vi "AmplifierPowerTest.vi"() -> ()   [LabVIEW 2020]
uses:
  FunctionVi/Window/Control/Channel.ctl
  FunctionVi/Queue/Control/QueueState.ctl
  FunctionVi/Window/Control/Bit rate.ctl
  FunctionVi/Window/Control/HwType.ctl
  FunctionVi/Window/Control/Mode.ctl
  <vilib>/Utility/xml.llb/Read From XML File(string).vi
  <vilib>/Utility/file.llb/Write Delimited Spreadsheet (string).vi
  <vilib>/Utility/xml.llb/Read From XML File(array).vi
  <vilib>/Utility/xml.llb/Write to XML File(string).vi
  <userlib>/FTLDCPower/MPD.lvlib
  <userlib>/PCAN-Basic/PCANBasic.lvlib
  FunctionVi/Window/Win_PowerAmplifier_Transmit.vi
panel:
  in  "USB Config":bool
  out "Interface Information: 3":string
  out "Elapsed Time (s)":dbl caption="已用时间(s)"
  out "Interface Information: 2":string
  in  "HostOCPEnable":bool
  in  "Host OCP":dbl caption="OCP:" format="%#.3gA"
  in  "HostOVPEnable":bool
  in  "Host OVP":dbl caption="OVP:" format="%#.3gV"
  in  "Host Current":dbl caption="Current:" format="%#.3gA"
  in  "Host Voltage":dbl caption="Voltage:" min=0.0 max=45.0 format="%#.3gV"
  out "Host Voltage out":dbl caption="Measure Voltage" format="%#.3gV"
  out "Host Power out":dbl caption="Measure Power" format="%#.3gW"
  out "Host Current out":dbl caption="Measure Current" format="%#.3gA"
  in  "Pause next(ms)":dbl=10.0 caption="Pause next:" min=10.0 format="%#.2fms"
  in  "Pause up(ms)":dbl=10.0 caption="Pause up:" format="%#.3fms"
  in  "ExecuteTime(s)":dbl=5.0 caption="Execute:" min=1.0 format="%#.3gs"
  out "x-y":u32
  out "Status":bool
  out "Company:":string
  out "Time:":string
  out "Channel:":T1 items=["PCAN_USBBUS1"=81, "PCAN_USBBUS2"=82, "PCAN_USBBUS3"=83, "PCAN_USBBUS4"=84]
  in  "PCAN Read error":string
  in  "source":string
  out "Status:":string
  out "Interface Information:":string
  in  "Max voltage":dbl
  in  "At voltage":dbl
  in  "List record":i32(listbox)
  in  "Reset":bool
  in  "指示灯":bool
  in  "On/Off":bool
  in  "ACCOCPEnable":bool
  in  "ACC OCP":dbl caption="OCP:" format="%#.3gA"
  in  "ACCOVPEnable":bool
  in  "ACC OVP":dbl caption="OVP:" format="%#.3gV"
  in  "ACC Current":dbl caption="Current:" min=0.0 format="%#.3gA"
  in  "ACC Voltage":dbl caption="Voltage:" min=0.0 max=45.0 format="%#.3gV"
  in  "Transmit info":bool
  in  "Receive":i32(listbox)
  out "LastError":string
  in  "PCAN Config":bool
  out "ACC Voltage out":dbl caption="Measure Voltage" format="%#.3gV"
  out "ACC Power out":dbl caption="Measure Power" format="%#.3gW"
  out "ACC Current out":dbl caption="Measure Current" format="%#.3gA"
  in  "RS232 Config":bool
  # "ACC Power"
  # "Host Power"
  # "Params Set"
  # "Measurement"
  # "Time"
  # "Output"
  # "Params Set"
  # "Measurement"
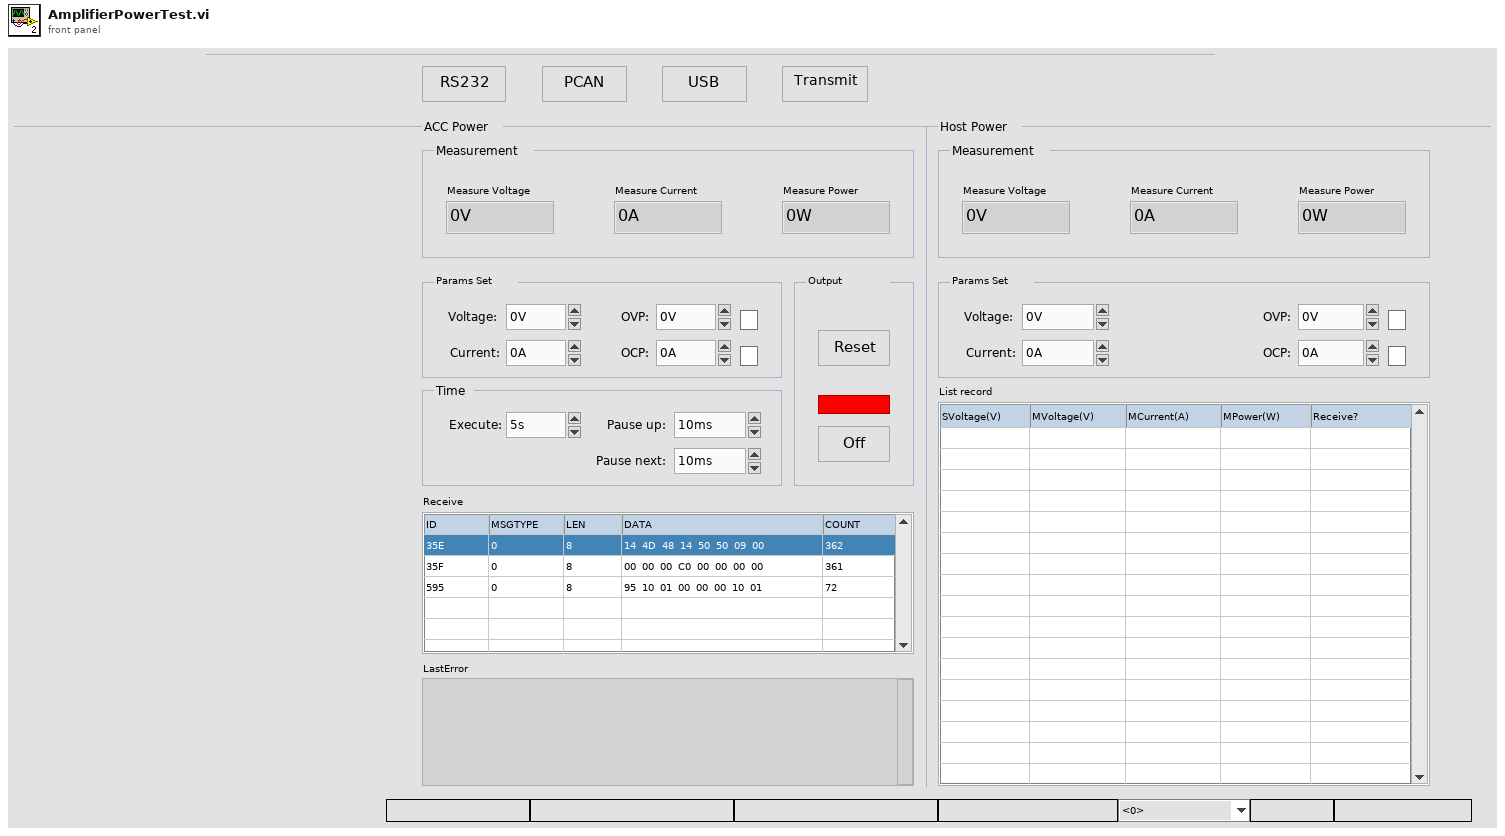
[diagram p1: front panel]
types:
  T1 = typedef "Channel.ctl" = u16
  T2 = typedef "QueueState.ctl" = enum16{"", "Create", "In", "Out", "Empty", "Close"}
  T3 = cluster{"ID":u32, "MSGTYPE":u8, "LEN":u8, "DATA[0]":u8, "DATA[1]":u8, "DATA[2]":u8, "DATA[3]":u8, "DATA[4]":u8, "DATA[5]":u8, "DATA[6]":u8, "DATA[7]":u8}
  T4 = enum8{"Enabled", "Disabled", "Disabled and Grayed Out"}
  T5 = cluster{"ACCCommName":refnum<visa-resource-name>, "HostCommName":refnum<visa-resource-name>}
  T6 = cluster{"ACC Serial Configuration":cluster{"Baud Rate":u32, "Parity":u16, "Data Bits":u16, "Stop Bits":u16, "Flow Control":u16}, "Host ACC Serial Configuration":cluster{"Baud Rate":u32, "Parity":u16, "Data Bits":u16, "Stop Bits":u16, "Flow Control":u16}}
  T7 = typedef "Mode.ctl" = u8
  T8 = typedef "Bit rate.ctl" = u16
  T9 = typedef "HwType.ctl" = u8
  T10 = enum16{"VOLTage", "DEFault", "MINimum", "MAXimum"}
  T11 = cluster{"Baud Rate":u32, "Parity":u16, "Data Bits":u16, "Stop Bits":u16, "Flow Control":u16}
  T12 = enum16{"current", "DEFault", "MINimum", "MAXimum"}
  T13 = typedef "LVPoint32TypeDef.ctl" = cluster{"Horizontal":i32, "Vertical":i32}
  T14 = typedef "LVRowAndColumnTypeDef.ctl" = cluster{"Row":i32, "Column":i32}
  T15 = cluster{"ID":u32, "MSGTYPE":u8, "LEN":u8, "DATA[0]":u8, "DATA[1]":u8, "DATA[2]":u8, "DATA[3]":u8, "DATA[4]":u8, "DATA[5]":u8, "DATA[6]":u8, "DATA[7]":u8}[]
  T16 = cluster{"Time":u16, "MessageBuffer":cluster{"ID":u32, "MSGTYPE":u8, "LEN":u8, "DATA[0]":u8, "DATA[1]":u8, "DATA[2]":u8, "DATA[3]":u8, "DATA[4]":u8, "DATA[5]":u8, "DATA[6]":u8, "DATA[7]":u8}[]}[]
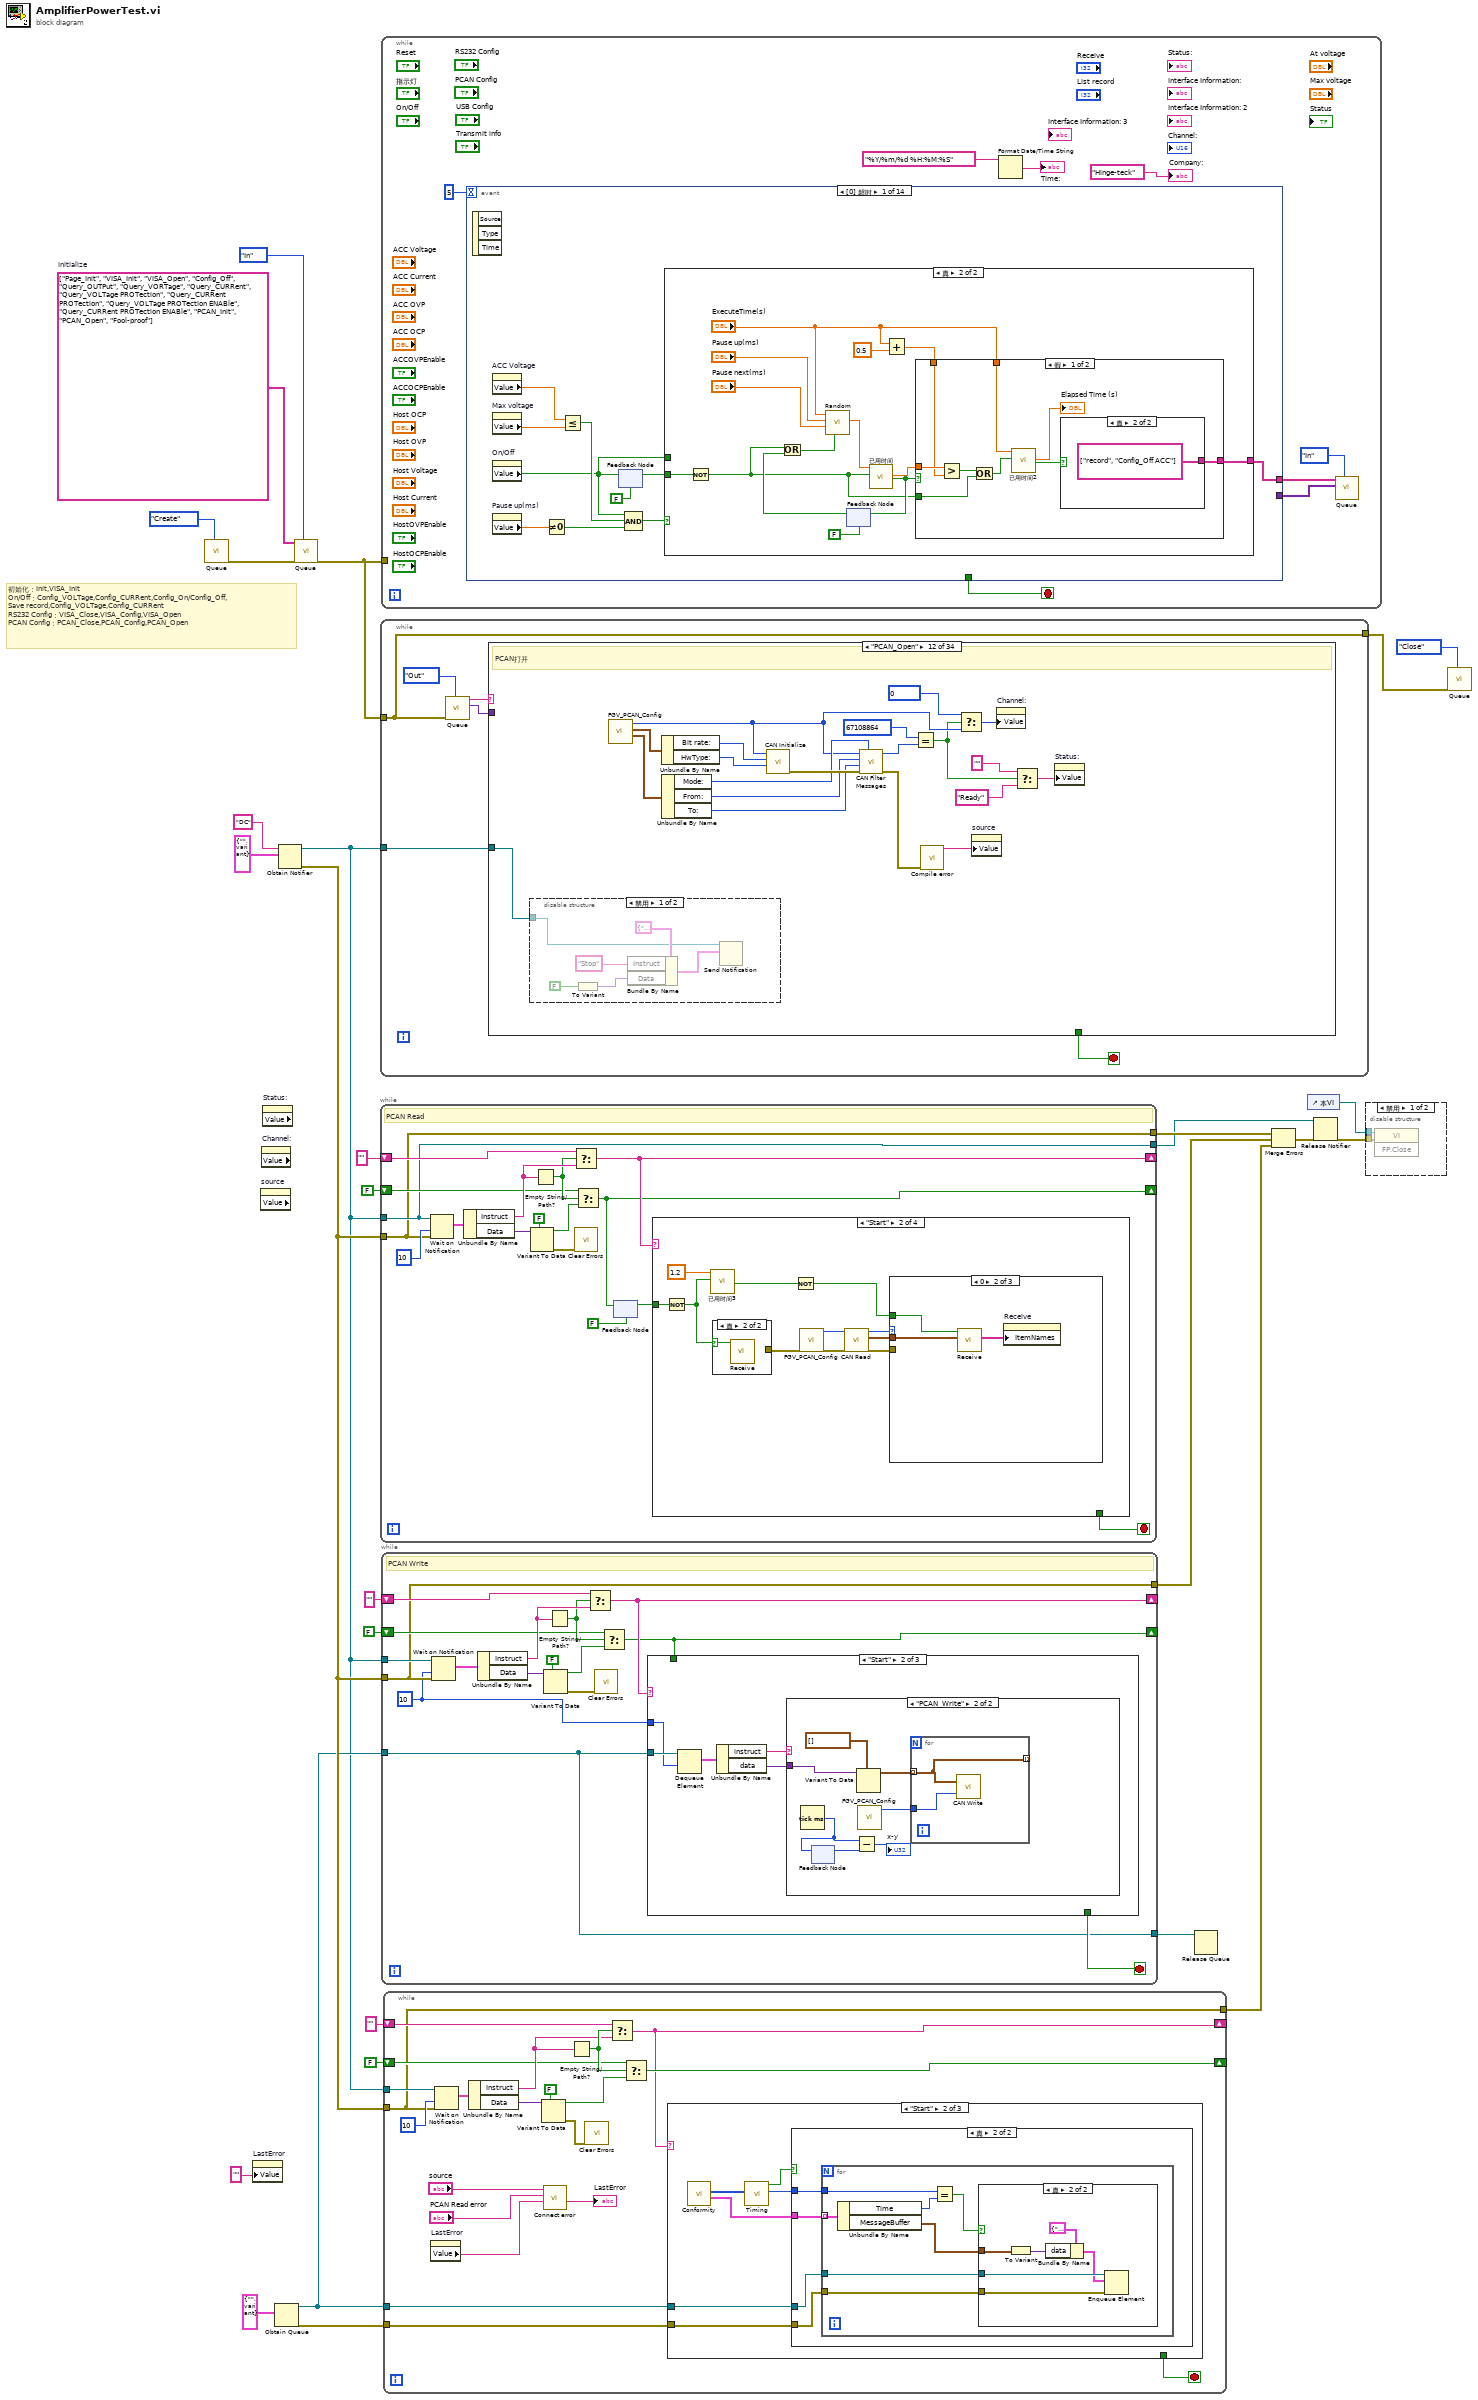
[diagram p0: block diagram]
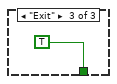
[diagram p6: hidden frame]
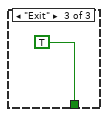
[diagram p9: hidden frame]
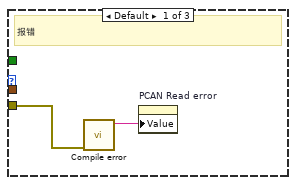
[diagram p11: hidden frame]
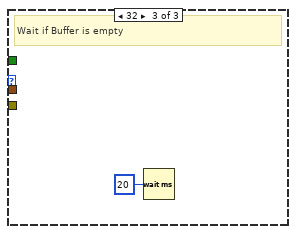
[diagram p12: hidden frame]
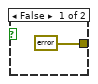
[diagram p13: hidden frame]
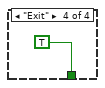
[diagram p15: hidden frame]
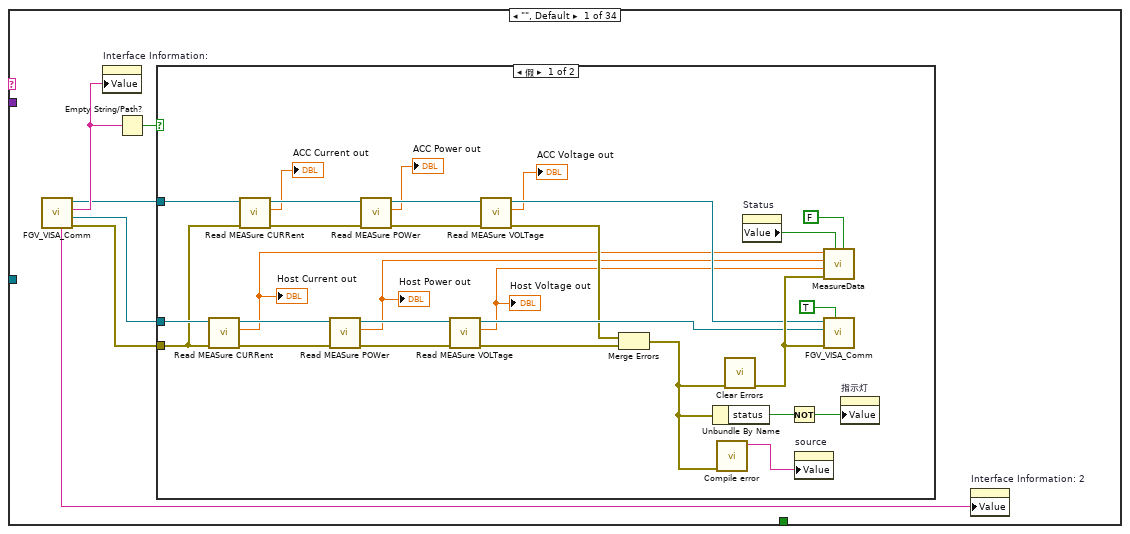
[diagram p16: hidden frame]
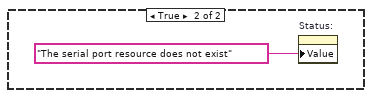
[diagram p17: hidden frame]
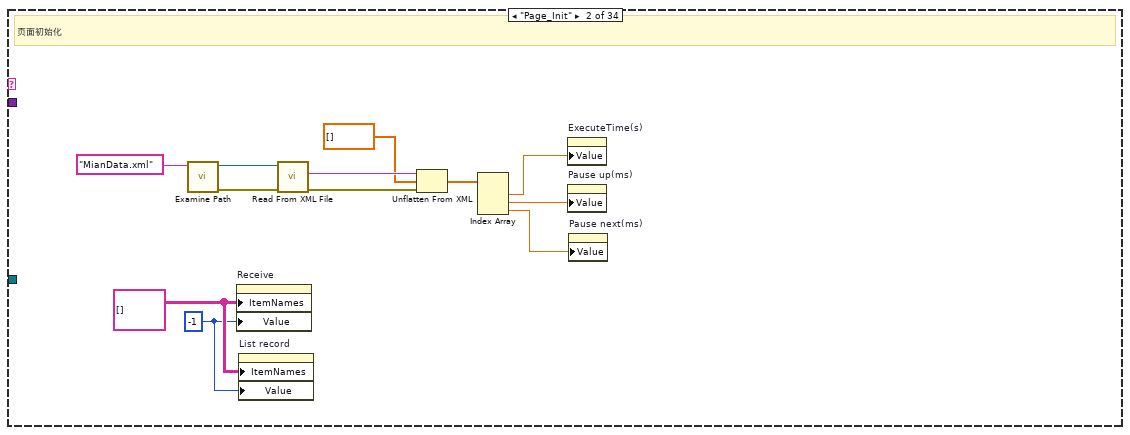
[diagram p18: hidden frame]
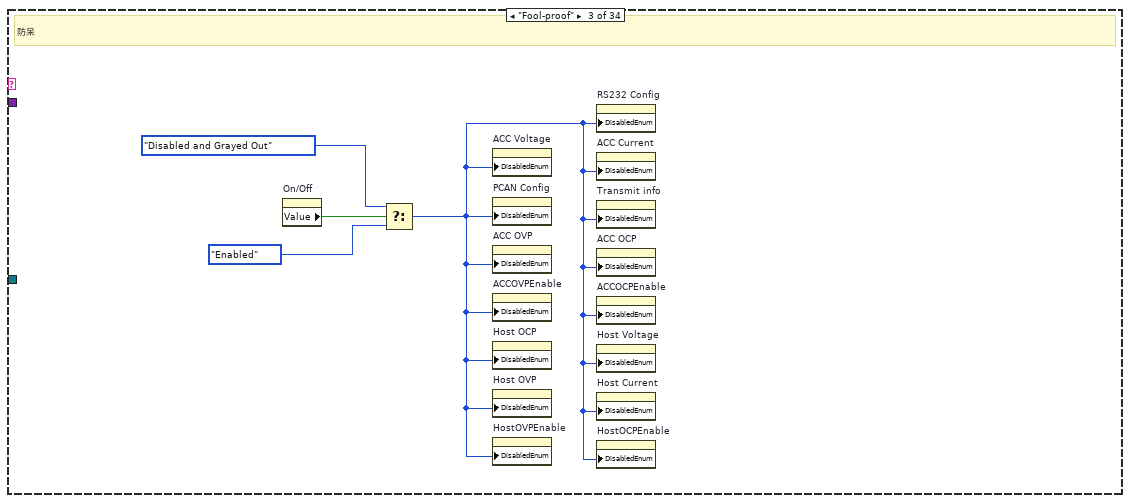
[diagram p19: hidden frame]
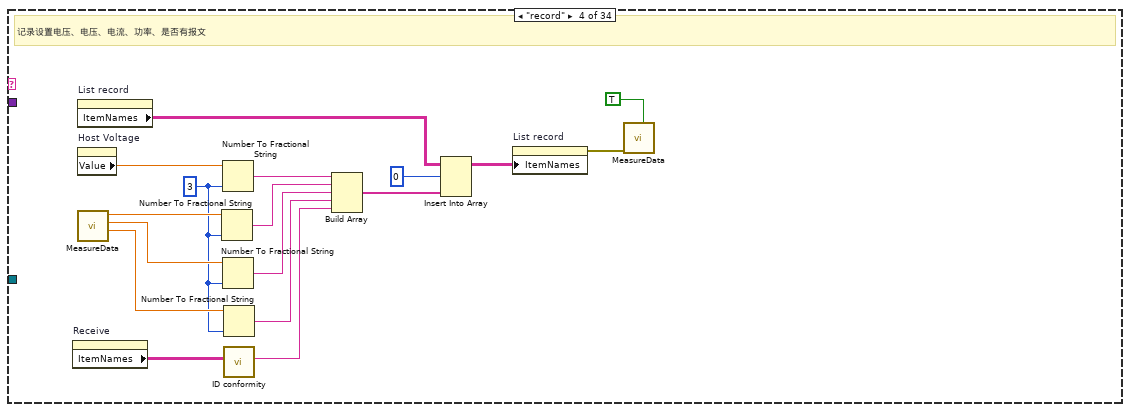
[diagram p20: hidden frame]
diagram:
  w25 = string[] ["Page_Init", "VISA_Init", "VISA_Open", "Config_Off", "Query_OUTPut", "Query_VORTage", "Query_CURRent", "Query_VOLTage PROTection", "Query_CURRent PROTection", "Query_VOLTage PROTection ENABle", "Query_CURRent PROTection ENABle", "PCAN_Init", "PCAN_Open", "Fool-proof"]  # Initialize
  # "初始化：Init,VISA_Init\nOn/Off：Config_VOLTage,Config_CURRent,Config_On/Config_Off,\nSave record,Config_VOLTage,Config_CURRent\nRS232 Config：VISA_Close,VISA_Config,VISA_Open\nPCAN Config：PCAN_Close,PCAN_Config,PCAN_Open"
  n1 = call "Queue.vi"("State"=QueueState."Create") -> ("error out"=w28:errorcluster)  [unwired: 8 in, 2 out]
  n2 = property on="LastError" class="Str"("Value"="") -> ()  [unwired: 2 in, 2 out]
  n3 = property on="source" class="Str" props=["Value"]() -> ()  [unwired: 2 in, 3 out]
  n4 = property on="Channel:" class="Ring (严格)" props=["Value"]() -> ()  [unwired: 2 in, 3 out]
  n5 = property on="Status:" class="Str" props=["Value"]() -> ()  [unwired: 2 in, 3 out]
  n6 = Obtain Queue(element data type=cluster{"instruct":string, "data":variant} {"instruct"="", "data"=variant}) -> (queue out=w19:refnum<queue>, error out=w6:errorcluster)  [unwired: 4 in, 1 out]
  n7 = Obtain Notifier(name (unnamed)="DC" ("名称（未命名）"), notification data type=cluster{"Instruct":string, "Data":variant} {"Instruct"="", "Data"=variant}) -> (notifier out=w18:refnum<notifier>, error out=w20:errorcluster)  [unwired: 2 in, 1 out]
  n8 = call "Queue.vi"("State"=QueueState."In", "error in"=w28, "Instruct"=w25) -> ("error out"=w27:errorcluster)  [unwired: 6 in, 2 out]
  n9 = while {
    tunnel: w20 -> [w30]
    tunnel: w18 -> [w35]
    shift-right: [w37] -> _
    shift-left: "" ("Instruct") -> [w43]
    shift-right: [w33] -> _
    shift-left: FALSE -> [w38]
    tunnel: [w35] -> w12
    tunnel: [w30] -> w14
    stop <- w36 stop-if-true
    # "PCAN Read"
    n10 = Wait on Notification(notifier=w35, timeout in ms (-1)=10 ("超时毫秒(-1)"), error in (no error)=w30) -> (notification=w45:cluster{"Instruct":string, "Data":variant})  [unwired: 1 in, 3 out]
    n11 = Unbundle By Name(w45) -> ("Instruct"=w44:string, "Data"=w41:variant)
    n12 = Variant To Data(type=FALSE, Variant=w41) -> (data=w39:bool, error out=w34:errorcluster)  [unwired: 1 in]
    n13 = Empty String/Path?(string/path=w44) -> (empty?=w42:bool)
    n14 = Select(t=w43, s=w42, f=w44) -> (s? t:f=w37:string)
    n15 = call <vilib>:"Clear Errors.vi"("error in (no error)"=w34) -> ()  [unwired: 5 in, 2 out]
    n16 = Select(t=w38, s=w42, f=w39) -> (s? t:f=w33:bool)
    n17 = feedback-in #1(w33) -> ()
    n18 = feedback #1(FALSE) -> (w31:bool)
    n19 = case shown="\"Start\"" w37 {
      tunnel: [_ _ _ TRUE] -> w36
      tunnel: w31 -> [_ w57 _ _]
      frame "假", Default {
      }
      frame "Start" {
        n20 = Not(x=w57) -> (.not. x?=w55:bool)
        n21 = call "已用时间3"("Time Target (s)"=1.2, "Reset"=w55) -> ("Time has Elapsed"=w48:bool)  [unwired: 10 in, 7 out]
        n22 = case shown="真" w55 {
          selector: w55 -> [_ w65]
          tunnel: [errorcluster {"status"=FALSE, "code"=0, "source"=""} ("错误常量") _] -> w56
          frame False {
          }
          frame True {
            n23 = call "Receive.vi"("Clear?"=w65) -> ()  [unwired: 10 in, 1 out]
          }
        }
        n24 = Not(x=w48) -> (.not. x?=w47:bool)
        n25 = call "FGV_PCAN_Config.vi"("error in"=w56) -> ("error out"=w51:errorcluster, "Channel out"=w53:T1)  [unwired: 7 in, 2 out]
        n26 = call <userlib>:"CAN Read.vi"("error in (no error)"=w51, "Channel"=w53) -> ("error out"=w50:errorcluster, "MessageBuffer out"=w49:T3, "function return"=w52:u32)  [unwired: 6 in, 1 out]
        n27 = case shown="0" w52 {
          tunnel: w50 -> [w59 _ _]
          tunnel: w49 -> [_ w62 _]
          tunnel: w47 -> [_ w60 _]
          frame Default {
            # "报错"
            n28 = call "Compile error.vi"("错误输入"=w59) -> ("Error out"=w58:string)  [unwired: 10 in]
            n29 = property on="PCAN Read error" class="Str"("Value"=w58) -> ()  [unwired: 2 in, 2 out]
          }
          frame 0 {
            n30 = call "Receive.vi"("MessageBuffer"=w62, "Clear?"=w60) -> ("Receive"=w61:string[][])  [unwired: 9 in]
            n31 = property on="Receive" class="MCListbox (严格)"("ItemNames"=w61) -> ()  [unwired: 2 in, 2 out]
          }
          frame 32 {
            # "Wait if Buffer is empty"
            n32 = Wait (ms)(milliseconds to wait=u32 20 ("等待时间（毫秒）")) -> ()  [unwired: 1 out]
          }
        }
      }
      frame "Stop" {
      }
      frame "Exit" {
      }
    }
  }
  n33 = while {
    tunnel: w27 -> [w68]
    tunnel: w18 -> [w67]
    tunnel: [w68] -> w22
    stop <- w70 stop-if-true
    n34 = call "Queue.vi"("State"=QueueState."Out", "error in"=w68) -> ("Data Out"=w69:variant, "Instruct Out"=w71:string)  [unwired: 7 in, 1 out]
    n35 = case shown="\"PCAN_Open\"" w71 {
      tunnel: [_ _ _ _ _ _ _ _ _ _ _ _ _ _ _ _ _ _ _ _ _ _ _ _ _ _ _ _ _ _ _ _ _ TRUE] -> w70
      tunnel: w69 -> [_ _ _ _ _ _ _ _ _ _ _ _ _ _ _ w280 _ _ _ _ _ _ _ _ _ _ _ _ _ _ _ _ _ _]
      tunnel: w67 -> [_ _ _ _ _ _ _ _ _ _ _ w236 _ _ _ _ _ _ _ _ _ w361 w375 w390 w406 w441 _ _ _ _ _ _ _ w548]
      frame "", Default {
        n36 = call "FGV_VISA_Comm.vi"() -> ("error out"=w78:errorcluster, "Host VISA resource name out"=w74:refnum<visa-resource-name>, "ACC Interface Information"=w76:string, "ACC VISA resource name out"=w73:refnum<visa-resource-name>, "Host Interface Information"=w75:string)  [unwired: 7 in]
        n37 = property on="Interface Information:" class="Str"("Value"=w76) -> ()  [unwired: 2 in, 2 out]
        n38 = Empty String/Path?(string/path=w76) -> (empty?=w77:bool)
        n39 = case shown="假" w77 {
          tunnel: w78 -> [w93 _]
          tunnel: w74 -> [w103 _]
          tunnel: w73 -> [w92 _]
          frame False {
            n40 = call <userlib>:"Read MEASure CURRent.vi"("error in (no error)"=w93, "VISA resource name"=w103) -> ("error out"=w107:errorcluster, "Measure Current"=w84:dbl, "VISA resource name out"=w104:refnum<visa-resource-name>)  [unwired: 7 in]
            "Host Current out" <- w84
            n41 = call <userlib>:"Read MEASure CURRent.vi"("error in (no error)"=w93, "VISA resource name"=w92) -> ("error out"=w94:errorcluster, "Measure Current"=→"ACC Current out":dbl, "VISA resource name out"=w91:refnum<visa-resource-name>)  [unwired: 7 in]
            n42 = call <userlib>:"Read MEASure POWer.vi"("error in (no error)"=w107, "VISA resource name"=w104) -> ("error out"=w105:errorcluster, "Measure Power"=w83:dbl, "VISA resource name out"=w106:refnum<visa-resource-name>)  [unwired: 7 in]
            "Host Power out" <- w83
            n43 = call <userlib>:"Read MEASure POWer.vi"("error in (no error)"=w94, "VISA resource name"=w91) -> ("error out"=w95:errorcluster, "Measure Power"=→"ACC Power out":dbl, "VISA resource name out"=w90:refnum<visa-resource-name>)  [unwired: 7 in]
            n44 = call <userlib>:"Read MEASure VOLTage.vi"("error in (no error)"=w105, "VISA resource name"=w106) -> ("error out"=w87:errorcluster, "Measure VOLTage"=w82:dbl, "VISA resource name out"=w88:refnum<visa-resource-name>)  [unwired: 7 in]
            "Host Voltage out" <- w82
            n45 = call <userlib>:"Read MEASure VOLTage.vi"("error in (no error)"=w95, "VISA resource name"=w90) -> ("error out"=w86:errorcluster, "Measure VOLTage"=→"ACC Voltage out":dbl, "VISA resource name out"=w89:refnum<visa-resource-name>)  [unwired: 7 in]
            n46 = Merge Errors(w86, w87) -> (w85:errorcluster)
            n47 = Unbundle By Name(w85) -> ("status"=w101:bool)
            n48 = call "Compile error.vi"("错误输入"=w85) -> ("Error out"=w98:string)  [unwired: 10 in]
            n49 = call <vilib>:"Clear Errors.vi"("error in (no error)"=w85) -> ("error out"=w99:errorcluster)  [unwired: 5 in, 1 out]
            n50 = property on="Status" class="Bool (严格)"() -> ("Value"=w97:bool)  [unwired: 2 in, 2 out]
            n51 = Not(x=w101) -> (.not. x?=w100:bool)
            n52 = property on="source" class="Str"("Value"=w98) -> ()  [unwired: 2 in, 2 out]
            n53 = call "MeasureData.vi"("Reset?"=FALSE, "Write?"=w97, "error in"=w99, "Measure Voltage"=w82, "Measure Power"=w83, "Measure Current"=w84) -> ()  [unwired: 2 in, 4 out]
            n54 = call "FGV_VISA_Comm.vi"("Write?"=TRUE, "error in"=w99, "Host VISA resource name"=w88, "ACC VISA resource name"=w89) -> ()  [unwired: 3 in, 5 out]
            n55 = property on="指示灯" class="Bool (严格)"("Value"=w100) -> ()  [unwired: 2 in, 2 out]
          }
          frame True {
            n56 = property on="Status:" class="Str"("Value"="The serial port resource does not exist") -> ()  [unwired: 2 in, 2 out]
          }
        }
        n57 = property on="Interface Information: 2" class="Str"("Value"=w75) -> ()  [unwired: 2 in, 2 out]
      }
      frame "Page_Init" {
        w119 = -1 ("Receive")
        w120 = string[][] [] ("项名")
        # "页面初始化"
        n58 = call "Examine Path.vi"("Filename"="MianData.xml") -> ("error out"=w116:errorcluster, "Path"=w117:path)  [unwired: 9 in]
        n59 = property on="Receive" class="MCListbox (严格)"("ItemNames"=w120, "Value"=w119) -> ()  [unwired: 2 in, 2 out]
        n60 = property on="List record" class="MCListbox (严格)"("ItemNames"=w120, "Value"=w119) -> ()  [unwired: 2 in, 2 out]
        n61 = call-poly <vilib>:"Read From XML File.vi"("error in (no error)"=w116, "XML File Path"=w117) -> ("error out"=w114:errorcluster, "XML Elements"=w115:string)  [unwired: 7 in, 1 out]
        n62 = Unflatten From XML(xml string=w115, type=dbl[] [], error in (no error)=w114) -> (value=w112:dbl[])  [unwired: 1 out]
        n63 = Index Array(array=w112) -> (element #1=w111:dbl, element #2=w110:dbl, element #3=w109:dbl)  [unwired: 3 in]
        n64 = property on="ExecuteTime(s)" class="DigNum (严格)"("Value"=w111) -> ()  [unwired: 2 in, 2 out]
        n65 = property on="Pause up(ms)" class="DigNum (严格)"("Value"=w110) -> ()  [unwired: 2 in, 2 out]
        n66 = property on="Pause next(ms)" class="DigNum (严格)"("Value"=w109) -> ()  [unwired: 2 in, 2 out]
      }
      frame "Fool-proof" {
        # "防呆"
        n67 = property on="On/Off" class="Bool (严格)"() -> ("Value"=w124:bool)  [unwired: 2 in, 2 out]
        n68 = Select(t=T4."Disabled and Grayed Out" ("禁用"), s=w124, f=T4."Enabled") -> (s? t:f=w121:T4)
        n69 = property on="ACC Voltage" class="DigNum (严格)"("DisabledEnum"=w121) -> ()  [unwired: 2 in, 2 out]
        n70 = property on="PCAN Config" class="Bool"("DisabledEnum"=w121) -> ()  [unwired: 2 in, 2 out]
        n71 = property on="ACC OVP" class="DigNum (严格)"("DisabledEnum"=w121) -> ()  [unwired: 2 in, 2 out]
        n72 = property on="ACCOVPEnable" class="Bool (严格)"("DisabledEnum"=w121) -> ()  [unwired: 2 in, 2 out]
        n73 = property on="Host OCP" class="DigNum (严格)"("DisabledEnum"=w121) -> ()  [unwired: 2 in, 2 out]
        n74 = property on="Host OVP" class="DigNum (严格)"("DisabledEnum"=w121) -> ()  [unwired: 2 in, 2 out]
        n75 = property on="HostOVPEnable" class="Bool (严格)"("DisabledEnum"=w121) -> ()  [unwired: 2 in, 2 out]
        n76 = property on="RS232 Config" class="Bool"("DisabledEnum"=w121) -> ()  [unwired: 2 in, 2 out]
        n77 = property on="ACC Current" class="DigNum (严格)"("DisabledEnum"=w121) -> ()  [unwired: 2 in, 2 out]
        n78 = property on="Transmit info" class="Bool"("DisabledEnum"=w121) -> ()  [unwired: 2 in, 2 out]
        n79 = property on="ACC OCP" class="DigNum (严格)"("DisabledEnum"=w121) -> ()  [unwired: 2 in, 2 out]
        n80 = property on="ACCOCPEnable" class="Bool (严格)"("DisabledEnum"=w121) -> ()  [unwired: 2 in, 2 out]
        n81 = property on="Host Voltage" class="DigNum (严格)"("DisabledEnum"=w121) -> ()  [unwired: 2 in, 2 out]
        n82 = property on="Host Current" class="DigNum (严格)"("DisabledEnum"=w121) -> ()  [unwired: 2 in, 2 out]
        n83 = property on="HostOCPEnable" class="Bool (严格)"("DisabledEnum"=w121) -> ()  [unwired: 2 in, 2 out]
      }
      frame "record" {
        w126 = i16 3 ("精度(6)")
        # "记录设置电压、电压、电流、功率、是否有报文"
        n84 = property on="Receive" class="MCListbox (严格)"() -> ("ItemNames"=w141:string[][])  [unwired: 2 in, 2 out]
        n85 = property on="List record" class="MCListbox (严格)"() -> ("ItemNames"=w135:string[][])  [unwired: 2 in, 2 out]
        n86 = property on="Host Voltage" class="DigNum (严格)"() -> ("Value"=w125:dbl)  [unwired: 2 in, 2 out]
        n87 = call "MeasureData.vi"() -> ("PowerAverage(..10)"=w129:dbl, "CurrentAverage(..10)"=w130:dbl, "VoltageAverage(..10)"=w131:dbl)  [unwired: 8 in, 1 out]
        n88 = Number To Fractional String(number=w131, precision (6)=w126) -> (F-format string=w139:string)  [unwired: 2 in]
        n89 = Number To Fractional String(number=w125, precision (6)=w126) -> (F-format string=w140:string)  [unwired: 2 in]
        n90 = Number To Fractional String(number=w130, precision (6)=w126) -> (F-format string=w138:string)  [unwired: 2 in]
        n91 = Number To Fractional String(number=w129, precision (6)=w126) -> (F-format string=w137:string)  [unwired: 2 in]
        n92 = call "ID conformity.vi"("项名"=w141) -> ("ID conformity"=w136:string)  [unwired: 10 in]
        n93 = Build Array(w140, w139, w138, w137, w136) -> (w134:string[])
        n94 = Insert Into Array(array=w135, index (row)=0 ("索引 (行)"), new element=w134) -> (w132:string[][])  [unwired: 1 in]
        n95 = property on="List record" class="MCListbox (严格)"("ItemNames"=w132) -> (error out=w128:errorcluster)  [unwired: 2 in, 1 out]
        n96 = call "MeasureData.vi"("Reset?"=TRUE, "error in"=w128) -> ()  [unwired: 6 in, 4 out]
      }
      frame "Save record" {
        n97 = Format Date/Time String(time format string (%c)="%Y-%m-%d %H-%M-%S" ("时间格式字符串(%c)")) -> (date/time string=w155:string)  [unwired: 2 in]
        n98 = call <vilib>:"Application Directory.vi"() -> ("Application Directory"=w158:path)
        n99 = Concatenate Strings("Data\\" ("字符串"), w155, " List record.csv" ("字符串")) -> (w153:string)
        n100 = property on="List record" class="MCListbox (严格)"() -> ("ItemNames"=w143:string[][], "ColHdrString"=w152:string[])  [unwired: 2 in, 2 out]
        n101 = Build Path(base path=w158, name or relative path=w153) -> (appended path=w144:path)
        n102 = Strip Path(path=w144) -> (stripped path=w149:path)  [unwired: 1 out]
        n103 = call <vilib>:"Check if File or Folder Exists.vi"("path"=w149) -> ("error out"=w146:errorcluster, "file or folder exists?"=w148:bool, "dup path"=w147:path)  [unwired: 8 in]
        n104 = Empty Array?(array=w143) -> (empty?=w142:bool)
        n105 = Insert Into Array(array=w143, index (row)=0 ("索引 (行)"), new element=w152) -> (w150:string[][])  [unwired: 1 in]
        n106 = case shown="真" w148 {
          tunnel: w147 -> [w165 _]
          tunnel: w146 -> [w164 w166]
          tunnel: [w163 w166] -> w145
          frame False {
            n107 = Create Folder(path (use dialog)=w165, error in=w164) -> (error out=w163:errorcluster)  [unwired: 1 in, 2 out]
          }
          frame True {
          }
        }
        n108 = case shown="真" w142 {
          tunnel: w150 -> [w161 _]
          tunnel: w145 -> [w160 _]
          tunnel: w144 -> [w159 _]
          frame False {
            n109 = call-poly <vilib>:"Write Delimited Spreadsheet.vi"("file path (dialog if empty)"=w159, "2D data"=w161, "error in (no error)"=w160, "delimiter (\\t)"="," ("delimiter (\\t)")) -> ()  [unwired: 10 in, 2 out]
          }
          frame True {
          }
        }
      }
      frame "VISA_Init" {
        # "VISA初始化"
        n110 = call "Examine Path.vi"("Filename"="RS232Data.xml") -> ("error out"=w174:errorcluster, "Path"=w175:path)  [unwired: 9 in]
        n111 = call-poly <vilib>:"Read From XML File.vi"("error in (no error)"=w174, "XML File Path"=w175) -> ("XML Elements"=w173:string[])  [unwired: 7 in, 2 out]
        n112 = Index Array(array=w173) -> (element #1=w172:string, element #2=w171:string)  [unwired: 2 in]
        n113 = Unflatten From XML(xml string=w171, type=T6 {"ACC Serial Configuration"={"Baud Rate"=9600, "Parity"=0, "Data Bits"=8, "Stop Bits"=10, "Flow Control"=0}, "Host ACC Serial Configuration"={"Baud Rate"=9600, "Parity"=0, "Data Bits"=8, "Stop Bits"=10, "Flow Control"=0}} ("Serial Configuration Out")) -> (value=w167:T6)  [unwired: 1 in, 1 out]
        n114 = Unflatten From XML(xml string=w172, type=T5 {"ACCCommName"="COM4", "HostCommName"="COM4"} ("CommNameOut")) -> (value=w168:T5)  [unwired: 1 in, 1 out]
        n115 = call "FGV_VISA_Config.vi"("Write?"=TRUE, "Serial Configuration"=w167, "CommName"=w168) -> ()  [unwired: 6 in, 3 out]
      }
      frame "VISA_Config" {
        # "VISA配置参数"
        n116 = call-by-ref "?"() -> ("Yes out"=w178:bool)  [unwired: 12 in, 3 out]
        n117 = case shown="真" w178 {
          frame False {
          }
          frame True {
            n118 = vi-ref "Win_RS232_Config.vi"() -> (w180:refnum<vi>)
            n119 = invoke class="VI" method="Default Vals.Make Curr Default"(reference=w180) -> (reference out=w179:refnum<vi>)  [unwired: 2 in, 2 out]
            n120 = Close Reference(reference=w179) -> ()  [unwired: 1 in, 1 out]
          }
        }
      }
      frame "VISA_Open" {
        w187 = refnum<visa-resource-name> refnum ("VISA resource name")
        # "VISA连接"
        n121 = call "FGV_VISA_Config.vi"() -> ("error out"=w193:errorcluster, "Serial Configuration Out"=w183:T6, "CommNameOut"=w196:T5)  [unwired: 9 in]
        n122 = Unbundle By Name(w196) -> ("ACCCommName"=w192:refnum<visa-resource-name>, "HostCommName"=w191:refnum<visa-resource-name>)
        n123 = Unbundle By Name(w183) -> ("ACC Serial Configuration"=w182:T11, "Host ACC Serial Configuration"=w181:T11)
        n124 = call <userlib>:"Close.vi"("error in (no error)"=w193, "VISA resource name"=w192) -> ("error out"=w205:errorcluster)  [unwired: 9 in]
        n125 = call <userlib>:"Close.vi"("error in (no error)"=w193, "VISA resource name"=w191) -> ("error out"=w194:errorcluster)  [unwired: 9 in]
        n126 = call <vilib>:"Clear Errors.vi"("error in (no error)"=w205) -> ("error out"=w204:errorcluster)  [unwired: 5 in, 1 out]
        n127 = call <vilib>:"Clear Errors.vi"("error in (no error)"=w194) -> ("error out"=w195:errorcluster)  [unwired: 5 in, 1 out]
        n128 = call <userlib>:"Initialize.vi"("VISA resource name"=w192, "Serial Configuration"=w182, "error in (no error)"=w204) -> ("VISA resource name out"=w199:refnum<visa-resource-name>, "error out"=w190:errorcluster)  [unwired: 6 in]
        n129 = call <userlib>:"Initialize.vi"("VISA resource name"=w191, "Serial Configuration"=w181, "error in (no error)"=w195) -> ("VISA resource name out"=w186:refnum<visa-resource-name>, "error out"=w189:errorcluster)  [unwired: 6 in]
        n130 = Merge Errors(w190, w189) -> (w184:errorcluster)
        n131 = Unbundle By Name(w184) -> ("code"=w202:i32)
        n132 = call "Compile error.vi"("错误输入"=w184) -> ("Error out"=w197:string)  [unwired: 10 in]
        n133 = Equal?(x=w202, y=-1073807343) -> (x = y?=w188:bool)
        n134 = property on="source" class="Str"("Value"=w197) -> ()  [unwired: 2 in, 2 out]
        n135 = Select(t=w187, s=w188, f=w199) -> (s? t:f=w198:refnum<visa-resource-name>)
        n136 = Select(t=w187, s=w188, f=w186) -> (s? t:f=w185:refnum<visa-resource-name>)
        n137 = case shown="真" w188 {
          frame False {
          }
          frame True {
            n138 = call "Queue.vi"("State"=QueueState."Empty") -> ()  [unwired: 8 in, 3 out]
          }
        }
        n139 = call "FGV_VISA_Comm.vi"("Write?"=TRUE, "error in"=w184, "Host VISA resource name"=w185, "ACC VISA resource name"=w198) -> ("error out"=w203:errorcluster)  [unwired: 3 in, 4 out]
        n140 = call <vilib>:"Clear Errors.vi"("error in (no error)"=w203) -> ()  [unwired: 5 in, 2 out]
      }
      frame "VISA_Close" {
        # "VISA关闭连接"
        n141 = call "FGV_VISA_Comm.vi"() -> ("error out"=w208:errorcluster, "Host VISA resource name out"=w207:refnum<visa-resource-name>, "ACC VISA resource name out"=w211:refnum<visa-resource-name>)  [unwired: 7 in, 2 out]
        n142 = call <userlib>:"Close.vi"("error in (no error)"=w208, "VISA resource name"=w211) -> ("error out"=w210:errorcluster)  [unwired: 9 in]
        n143 = call <userlib>:"Close.vi"("error in (no error)"=w208, "VISA resource name"=w207) -> ("error out"=w209:errorcluster)  [unwired: 9 in]
        n144 = call <vilib>:"Clear Errors.vi"("error in (no error)"=w210) -> ()  [unwired: 5 in, 2 out]
        n145 = call <vilib>:"Clear Errors.vi"("error in (no error)"=w209) -> ()  [unwired: 5 in, 2 out]
      }
      frame "PCAN_Init" {
        w219 = T1 81 items=["PCAN_USBBUS1"=81, "PCAN_USBBUS2"=82, "PCAN_USBBUS3"=83, "PCAN_USBBUS4"=84] ("Channel:")
        # "PCAN读取配置"
        n146 = call "Examine Path.vi"("Filename"="PCANData.xml") -> ("error out"=w222:errorcluster, "Path"=w223:path)  [unwired: 9 in]
        n147 = call-poly <vilib>:"Read From XML File.vi"("error in (no error)"=w222, "XML File Path"=w223) -> ("XML Elements"=w221:string[])  [unwired: 7 in, 2 out]
        n148 = call "Examine Path.vi"("Filename"="TransmitData.xml") -> ("error out"=w229:errorcluster, "Path"=w230:path)  [unwired: 9 in]
        n149 = Index Array(array=w221) -> (element #1=w220:string, element #2=w217:string, element #3=w214:string)  [unwired: 3 in]
        n150 = call-poly <vilib>:"Read From XML File.vi"("error in (no error)"=w229, "XML File Path"=w230) -> ("XML Elements"=w228:string)  [unwired: 7 in, 2 out]
        n151 = Unflatten From XML(xml string=w220, type=w219) -> (value=w218:T1)  [unwired: 1 in, 1 out]
        n152 = Unflatten From XML(xml string=w228, type=string[][] []) -> (value=w226:string[][])  [unwired: 1 in, 1 out]
        n153 = Unflatten From XML(xml string=w217, type=cluster{"Bit rate:":T8, "HwType: ":T9} {"Bit rate:"=28, "HwType: "=1} ("Initialize")) -> (value=w215:cluster{"Bit rate:":T8, "HwType: ":T9})  [unwired: 1 in, 1 out]
        n154 = Unflatten From XML(xml string=w214, type=cluster{"Mode: ":T7, "From:":u32, "To:":u32} {"Mode: "=0, "From:"=0, "To:"=0} ("FilterMessages")) -> (value=w212:cluster{"Mode: ":T7, "From:":u32, "To:":u32})  [unwired: 1 in, 1 out]
        n155 = call "FGV_PowerAmplifier_Transmit.vi"("Write?"=TRUE, "Transmit"=w226) -> ()  [unwired: 8 in, 2 out]
        n156 = call "FGV_PCAN_Config.vi"("Write?"=TRUE, "FilterMessages"=w212, "Initialize"=w215, "Channel"=w218) -> ()  [unwired: 4 in, 4 out]
      }
      frame "PCAN_Config" {
        # "PCAN配置"
        n157 = call-by-ref "?"() -> ("Yes out"=w233:bool)  [unwired: 9 in, 6 out]
        n158 = case shown="真" w233 {
          frame False {
          }
          frame True {
            n159 = vi-ref "Win_PCAN_Config.vi"() -> (w235:refnum<vi>)
            n160 = invoke class="VI" method="Default Vals.Make Curr Default"(reference=w235) -> (reference out=w234:refnum<vi>)  [unwired: 2 in, 2 out]
            n161 = Close Reference(reference=w234) -> ()  [unwired: 1 in, 1 out]
          }
        }
      }
      frame "PCAN_Open" {
        w242 = T1 0 items=["PCAN_USBBUS1"=81, "PCAN_USBBUS2"=82, "PCAN_USBBUS3"=83, "PCAN_USBBUS4"=84] ("t")
        # "PCAN打开"
        n162 = disable-structure shown="禁用" {
          disable-tunnel: w236 -> [w256 _]
          frame Disabled {
            n163 = To Variant(anything=FALSE) -> (Variant=w258:variant)
            n164 = Bundle By Name(cluster=cluster{"Instruct":string, "Data":variant} {"Instruct"="", "Data"=variant}, "Instruct"="Stop", "Data"=w258) -> (w261:cluster{"Instruct":string, "Data":variant})
            n165 = Send Notification(notification=w261, notifier=w256) -> ()  [unwired: 1 in, 2 out]
          }
          frame Enabled {
          }
        }
        n166 = call "FGV_PCAN_Config.vi"() -> ("FilterMessages out"=w254:cluster{"Mode: ":T7, "From:":u32, "To:":u32}, "Initialize out"=w255:cluster{"Bit rate:":T8, "HwType: ":T9}, "Channel out"=w243:T1)  [unwired: 8 in, 1 out]
        n167 = Unbundle By Name(w255) -> ("Bit rate:"=w253:T8, "HwType:"=w252:T9)
        n168 = Unbundle By Name(w254) -> ("Mode:"=w250:T7, "From:"=w249:u32, "To:"=w248:u32)
        n169 = call <userlib>:"CAN Initialize.vi"("HwType"=w252, "Btr0Btr1"=w253, "Channel"=w243) -> ("错误输出"=w251:errorcluster)  [unwired: 7 in, 1 out]
        n170 = call <userlib>:"CAN Filter Messages.vi"("Mode"=w250, "error in (no error)"=w251, "ToID"=w248, "FromID"=w249, "Channel"=w243) -> ("error out"=w247:errorcluster, "function return"=w245:u32)  [unwired: 5 in]
        n171 = Equal?(x=u32 67108864, y=w245) -> (x = y?=w240:bool)
        n172 = call "Compile error.vi"("错误输入"=w247) -> ("Error out"=w246:string)  [unwired: 10 in]
        n173 = Select(t=w242, s=w240, f=w243) -> (s? t:f=w241:T1)
        n174 = property on="source" class="Str"("Value"=w246) -> ()  [unwired: 2 in, 2 out]
        n175 = property on="Channel:" class="Ring (严格)"("Value"=w241) -> ()  [unwired: 2 in, 2 out]
        n176 = Select(t="", s=w240, f="Ready") -> (s? t:f=w237:string)
        n177 = property on="Status:" class="Str"("Value"=w237) -> ()  [unwired: 2 in, 2 out]
      }
      frame "PCAN_Close" {
        # "PCAN关闭"
        n178 = call "FGV_PCAN_Config.vi"() -> ("Channel out"=w262:T1)  [unwired: 8 in, 3 out]
        n179 = call <userlib>:"CAN Uninitialize.vi"("Channel"=w262) -> ()  [unwired: 10 in, 1 out]
      }
      frame "Transmit_info" {
        # "报文"
        n180 = call-by-ref "?"() -> ("Yes out"=w263:bool)  [unwired: 12 in, 3 out]
        n181 = case shown="真" w263 {
          frame False {
          }
          frame True {
            n182 = vi-ref "Win_PCAN_Config.vi"() -> (w265:refnum<vi>)
            n183 = invoke class="VI" method="Default Vals.Make Curr Default"(reference=w265) -> (reference out=w264:refnum<vi>)  [unwired: 2 in, 2 out]
            n184 = Close Reference(reference=w264) -> ()  [unwired: 1 in, 1 out]
          }
        }
      }
      frame "Config_VOLTage" {
        # "设置输出电压"
        n185 = call "FGV_VISA_Comm.vi"() -> ("error out"=w272:errorcluster, "Host VISA resource name out"=w273:refnum<visa-resource-name>, "ACC VISA resource name out"=w278:refnum<visa-resource-name>)  [unwired: 7 in, 2 out]
        n186 = property on="Host Voltage" class="DigNum (严格)"() -> ("Value"=w271:dbl)  [unwired: 2 in, 2 out]
        n187 = property on="ACC Voltage" class="DigNum (严格)"() -> ("Value"=w275:dbl)  [unwired: 2 in, 2 out]
        n188 = call <userlib>:"Configure VOLTage LEVel.vi"("VOLTage  Value(V)"=w275, "error in (no error)"=w272, "VOLTage Tab"=T10."VOLTage", "VISA resource name"=w278) -> ("error out"=w269:errorcluster, "VISA resource name out"=w277:refnum<visa-resource-name>)  [unwired: 6 in]
        n189 = call <userlib>:"Configure VOLTage LEVel.vi"("VOLTage  Value(V)"=w271, "error in (no error)"=w272, "VOLTage Tab"=T10."VOLTage", "VISA resource name"=w273) -> ("error out"=w268:errorcluster, "VISA resource name out"=w270:refnum<visa-resource-name>)  [unwired: 6 in]
        n190 = Merge Errors(w269, w268) -> (w267:errorcluster)
        n191 = call "FGV_VISA_Comm.vi"("Write?"=TRUE, "error in"=w267, "Host VISA resource name"=w270, "ACC VISA resource name"=w277) -> ("error out"=w266:errorcluster)  [unwired: 3 in, 4 out]
        n192 = call <vilib>:"Clear Errors.vi"("error in (no error)"=w266) -> ()  [unwired: 5 in, 2 out]
      }
      frame "Config_VOLTage1" {
        # "设置输出电压"
        n193 = disable-structure shown="禁用" {
          disable-tunnel: w280 -> [w283 _]
          frame Disabled {
            n194 = Variant To Data(type=0.0 ("x+y"), Variant=w283) -> (data=w281:dbl)  [unwired: 1 in, 1 out]
            n195 = call "FGV_VISA_Comm.vi"() -> ("error out"=w286:errorcluster, "ACC VISA resource name out"=w288:refnum<visa-resource-name>)  [unwired: 7 in, 3 out]
            n196 = call <userlib>:"Configure VOLTage LEVel.vi"("VOLTage  Value(V)"=w281, "error in (no error)"=w286, "VOLTage Tab"=T10."VOLTage", "VISA resource name"=w288) -> ("error out"=w285:errorcluster, "VISA resource name out"=w287:refnum<visa-resource-name>)  [unwired: 6 in]
            n197 = call "FGV_VISA_Comm.vi"("Write?"=TRUE, "error in"=w285, "ACC VISA resource name"=w287) -> ()  [unwired: 4 in, 5 out]
          }
          frame Enabled {
          }
        }
      }
      frame "Config_CURRent" {
        w296 = T12."current" ("Current Tab")
        # "设置输出电流"
        n198 = call "FGV_VISA_Comm.vi"() -> ("error out"=w298:errorcluster, "Host VISA resource name out"=w295:refnum<visa-resource-name>, "ACC VISA resource name out"=w299:refnum<visa-resource-name>)  [unwired: 7 in, 2 out]
        n199 = property on="ACC Current" class="DigNum (严格)"() -> ("Value"=w297:dbl)  [unwired: 2 in, 2 out]
        n200 = property on="Host Current" class="DigNum (严格)"() -> ("Value"=w290:dbl)  [unwired: 2 in, 2 out]
        n201 = call <userlib>:"Configure CURRent LEVel.vi"("Current  Value(A)"=w297, "error in (no error)"=w298, "Current Tab"=w296, "VISA resource name"=w299) -> ("error out"=w293:errorcluster, "VISA resource name out"=w300:refnum<visa-resource-name>)  [unwired: 6 in]
        n202 = call <userlib>:"Configure CURRent LEVel.vi"("Current  Value(A)"=w290, "Current Tab"=w296, "VISA resource name"=w295) -> ("error out"=w292:errorcluster, "VISA resource name out"=w294:refnum<visa-resource-name>)  [unwired: 7 in]
        n203 = Merge Errors(w293, w292) -> (w291:errorcluster)
        n204 = call "FGV_VISA_Comm.vi"("Write?"=TRUE, "error in"=w291, "Host VISA resource name"=w294, "ACC VISA resource name"=w300) -> ()  [unwired: 3 in, 5 out]
      }
      frame "Config_VOLTage PROTection" {
        w307 = T10."VOLTage" ("VOLTage Tab")
        # "设置输出电压保护阈值"
        n205 = call "FGV_VISA_Comm.vi"() -> ("error out"=w308:errorcluster, "Host VISA resource name out"=w309:refnum<visa-resource-name>, "ACC VISA resource name out"=w311:refnum<visa-resource-name>)  [unwired: 7 in, 2 out]
        n206 = property on="ACC OVP" class="DigNum (严格)"() -> ("Value"=w310:dbl)  [unwired: 2 in, 2 out]
        n207 = property on="Host OVP" class="DigNum (严格)"() -> ("Value"=w306:dbl)  [unwired: 2 in, 2 out]
        n208 = call <userlib>:"Configure VOLTage PROTection LEVel.vi"("VISA resource name"=w309, "VOLTage Tab"=w307, "VOLTage Protection Value(V)"=w306, "error in (no error)"=w308) -> ("VISA resource name out"=w305:refnum<visa-resource-name>, "error out"=w303:errorcluster)  [unwired: 4 in]
        n209 = call <userlib>:"Configure VOLTage PROTection LEVel.vi"("VISA resource name"=w311, "VOLTage Tab"=w307, "VOLTage Protection Value(V)"=w310, "error in (no error)"=w308) -> ("VISA resource name out"=w312:refnum<visa-resource-name>, "error out"=w304:errorcluster)  [unwired: 4 in]
        n210 = Merge Errors(w304, w303) -> (w302:errorcluster)
        n211 = call "FGV_VISA_Comm.vi"("Write?"=TRUE, "error in"=w302, "Host VISA resource name"=w305, "ACC VISA resource name"=w312) -> ()  [unwired: 3 in, 5 out]
      }
      frame "Config_CURRent PROTection" {
        w320 = T12."current" ("Current Tab")
        # "设置输出电流保护阈值"
        n212 = call "FGV_VISA_Comm.vi"() -> ("error out"=w319:errorcluster, "Host VISA resource name out"=w321:refnum<visa-resource-name>, "ACC VISA resource name out"=w323:refnum<visa-resource-name>)  [unwired: 7 in, 2 out]
        n213 = property on="ACC OCP" class="DigNum (严格)"() -> ("Value"=w322:dbl)  [unwired: 2 in, 2 out]
        n214 = property on="Host OCP" class="DigNum (严格)"() -> ("Value"=w318:dbl)  [unwired: 2 in, 2 out]
        n215 = call <userlib>:"Configure CURRent PROTection LEVel.vi"("VISA resource name"=w323, "Current Tab"=w320, "Current Protection Value(A)"=w322, "error in (no error)"=w319) -> ("VISA resource name out"=w324:refnum<visa-resource-name>, "error out"=w316:errorcluster)  [unwired: 4 in]
        n216 = call <userlib>:"Configure CURRent PROTection LEVel.vi"("VISA resource name"=w321, "Current Tab"=w320, "Current Protection Value(A)"=w318, "error in (no error)"=w319) -> ("VISA resource name out"=w317:refnum<visa-resource-name>, "error out"=w315:errorcluster)  [unwired: 4 in]
        n217 = Merge Errors(w316, w315) -> (w314:errorcluster)
        n218 = call "FGV_VISA_Comm.vi"("Write?"=TRUE, "error in"=w314, "Host VISA resource name"=w317, "ACC VISA resource name"=w324) -> ()  [unwired: 3 in, 5 out]
      }
      frame "Config_VOLTage PROTection ENABle" {
        # "禁止或使能当前输出电压保护电路"
        n219 = call "FGV_VISA_Comm.vi"() -> ("error out"=w331:errorcluster, "Host VISA resource name out"=w332:refnum<visa-resource-name>, "ACC VISA resource name out"=w334:refnum<visa-resource-name>)  [unwired: 7 in, 2 out]
        n220 = property on="HostOVPEnable" class="Bool (严格)"() -> ("Value"=w330:bool)  [unwired: 2 in, 2 out]
        n221 = property on="ACCOVPEnable" class="Bool (严格)"() -> ("Value"=w333:bool)  [unwired: 2 in, 2 out]
        n222 = call <userlib>:"Configure VOLTage PROTection ENABle.vi"("error in (no error)"=w331, "Enable VOLTage protection (T: Enable)"=w333, "VISA resource name"=w334) -> ("error out"=w328:errorcluster, "VISA resource name out"=w335:refnum<visa-resource-name>)  [unwired: 7 in]
        n223 = call <userlib>:"Configure VOLTage PROTection ENABle.vi"("error in (no error)"=w331, "Enable VOLTage protection (T: Enable)"=w330, "VISA resource name"=w332) -> ("error out"=w327:errorcluster, "VISA resource name out"=w329:refnum<visa-resource-name>)  [unwired: 7 in]
        n224 = Merge Errors(w328, w327) -> (w326:errorcluster)
        n225 = call "FGV_VISA_Comm.vi"("Write?"=TRUE, "error in"=w326, "Host VISA resource name"=w329, "ACC VISA resource name"=w335) -> ()  [unwired: 3 in, 5 out]
      }
      frame "Config_CURRent PROTection ENABle" {
        # "禁止或使能当前输出电压保护电路"
        n226 = call "FGV_VISA_Comm.vi"() -> ("error out"=w342:errorcluster, "Host VISA resource name out"=w343:refnum<visa-resource-name>, "ACC VISA resource name out"=w345:refnum<visa-resource-name>)  [unwired: 7 in, 2 out]
        n227 = property on="HostOCPEnable" class="Bool (严格)"() -> ("Value"=w341:bool)  [unwired: 2 in, 2 out]
        n228 = property on="ACCOCPEnable" class="Bool (严格)"() -> ("Value"=w344:bool)  [unwired: 2 in, 2 out]
        n229 = call <userlib>:"Configure CURRent PROTection ENABle.vi"("error in (no error)"=w342, "Enable Current protection (T: Enable)"=w344, "VISA resource name"=w345) -> ("error out"=w339:errorcluster, "VISA resource name out"=w346:refnum<visa-resource-name>)  [unwired: 7 in]
        n230 = call <userlib>:"Configure CURRent PROTection ENABle.vi"("error in (no error)"=w342, "Enable Current protection (T: Enable)"=w341, "VISA resource name"=w343) -> ("error out"=w338:errorcluster, "VISA resource name out"=w340:refnum<visa-resource-name>)  [unwired: 7 in]
        n231 = Merge Errors(w339, w338) -> (w337:errorcluster)
        n232 = call "FGV_VISA_Comm.vi"("Write?"=TRUE, "error in"=w337, "Host VISA resource name"=w340, "ACC VISA resource name"=w346) -> ()  [unwired: 3 in, 5 out]
      }
      frame "Config_On" {
        w353 = TRUE ("Enable OUTPut (T: Enable)")
        # "VISA打开通道"
        n233 = To Variant(anything=TRUE) -> (Variant=w356:variant)
        n234 = Bundle By Name(cluster=cluster{"Instruct":string, "Data":variant} {"Instruct"="", "Data"=variant} ("通知"), "Instruct"="Start", "Data"=w356) -> (w359:cluster{"Instruct":string, "Data":variant})
        n235 = call "FGV_VISA_Comm.vi"() -> ("error out"=w352:errorcluster, "Host VISA resource name out"=w354:refnum<visa-resource-name>, "ACC VISA resource name out"=w364:refnum<visa-resource-name>)  [unwired: 7 in, 2 out]
        n236 = Send Notification(notification=w359, notifier=w361) -> ()  [unwired: 1 in, 2 out]
        n237 = call <userlib>:"Configure OUTPut ENABle.vi"("error in (no error)"=w352, "Enable OUTPut (T: Enable)"=w353, "VISA resource name"=w364) -> ("error out"=w350:errorcluster, "VISA resource name out"=w363:refnum<visa-resource-name>)  [unwired: 7 in]
        n238 = call <userlib>:"Configure OUTPut ENABle.vi"("error in (no error)"=w352, "Enable OUTPut (T: Enable)"=w353, "VISA resource name"=w354) -> ("error out"=w349:errorcluster, "VISA resource name out"=w351:refnum<visa-resource-name>)  [unwired: 7 in]
        n239 = Merge Errors(w350, w349) -> (w348:errorcluster)
        n240 = call "FGV_VISA_Comm.vi"("Write?"=TRUE, "error in"=w348, "Host VISA resource name"=w351, "ACC VISA resource name"=w363) -> ()  [unwired: 3 in, 5 out]
        n241 = property on="Status" class="Bool (严格)"("Value"=TRUE ("Status")) -> ()  [unwired: 2 in, 2 out]
      }
      frame "Config_On ACC" {
        # "VISA打开通道"
        n242 = To Variant(anything=TRUE) -> (Variant=w370:variant)
        n243 = Bundle By Name(cluster=cluster{"Instruct":string, "Data":variant} {"Instruct"="", "Data"=variant} ("通知"), "Instruct"="Start", "Data"=w370) -> (w373:cluster{"Instruct":string, "Data":variant})
        n244 = call "FGV_VISA_Comm.vi"() -> ("error out"=w367:errorcluster, "Host VISA resource name out"=w365:refnum<visa-resource-name>, "ACC VISA resource name out"=w378:refnum<visa-resource-name>)  [unwired: 7 in, 2 out]
        n245 = Send Notification(notification=w373, notifier=w375) -> ()  [unwired: 1 in, 2 out]
        n246 = call <userlib>:"Configure OUTPut ENABle.vi"("error in (no error)"=w367, "Enable OUTPut (T: Enable)"=TRUE, "VISA resource name"=w378) -> ("error out"=w366:errorcluster, "VISA resource name out"=w377:refnum<visa-resource-name>)  [unwired: 7 in]
        n247 = call "FGV_VISA_Comm.vi"("Write?"=TRUE, "error in"=w366, "Host VISA resource name"=w365, "ACC VISA resource name"=w377) -> ()  [unwired: 3 in, 5 out]
        n248 = property on="Status" class="Bool (严格)"("Value"=TRUE ("Status")) -> ()  [unwired: 2 in, 2 out]
      }
      frame "Config_Off" {
        w385 = FALSE ("Enable OUTPut (T: Enable)")
        # "VISA关闭通道"
        n249 = To Variant(anything=FALSE) -> (Variant=w391:variant)
        n250 = Bundle By Name(cluster=cluster{"Instruct":string, "Data":variant} {"Instruct"="", "Data"=variant}, "Instruct"="Stop", "Data"=w391) -> (w394:cluster{"Instruct":string, "Data":variant})
        n251 = call "FGV_VISA_Comm.vi"() -> ("error out"=w383:errorcluster, "Host VISA resource name out"=w384:refnum<visa-resource-name>, "ACC VISA resource name out"=w397:refnum<visa-resource-name>)  [unwired: 7 in, 2 out]
        n252 = Send Notification(notification=w394, notifier=w390) -> ()  [unwired: 1 in, 2 out]
        n253 = call <userlib>:"Configure OUTPut ENABle.vi"("error in (no error)"=w383, "Enable OUTPut (T: Enable)"=w385, "VISA resource name"=w397) -> ("error out"=w381:errorcluster, "VISA resource name out"=w396:refnum<visa-resource-name>)  [unwired: 7 in]
        n254 = call <userlib>:"Configure OUTPut ENABle.vi"("error in (no error)"=w383, "Enable OUTPut (T: Enable)"=w385, "VISA resource name"=w384) -> ("error out"=w380:errorcluster, "VISA resource name out"=w382:refnum<visa-resource-name>)  [unwired: 7 in]
        n255 = Merge Errors(w381, w380) -> (w379:errorcluster)
        n256 = call <vilib>:"Clear Errors.vi"("error in (no error)"=w379) -> ("error out"=w388:errorcluster)  [unwired: 5 in, 1 out]
        n257 = call "Compile error.vi"("错误输入"=w379) -> ("Error out"=w387:string)  [unwired: 10 in]
        n258 = property on="source" class="Str"("Value"=w387) -> ()  [unwired: 2 in, 2 out]
        n259 = call "FGV_VISA_Comm.vi"("Write?"=TRUE, "error in"=w388, "Host VISA resource name"=w382, "ACC VISA resource name"=w396) -> ()  [unwired: 3 in, 5 out]
        n260 = property on="Status" class="Bool (严格)"("Value"=FALSE ("Status")) -> ()  [unwired: 2 in, 2 out]
      }
      frame "Config_Off ACC" {
        # "VISA关闭通道"
        n261 = To Variant(anything=FALSE) -> (Variant=w407:variant)
        n262 = Bundle By Name(cluster=cluster{"Instruct":string, "Data":variant} {"Instruct"="", "Data"=variant}, "Instruct"="Stop", "Data"=w407) -> (w410:cluster{"Instruct":string, "Data":variant})
        n263 = Send Notification(notification=w410, notifier=w406) -> ()  [unwired: 1 in, 2 out]
        n264 = call "FGV_VISA_Comm.vi"() -> ("error out"=w400:errorcluster, "Host VISA resource name out"=w398:refnum<visa-resource-name>, "ACC VISA resource name out"=w413:refnum<visa-resource-name>)  [unwired: 7 in, 2 out]
        n265 = call <userlib>:"Configure OUTPut ENABle.vi"("error in (no error)"=w400, "Enable OUTPut (T: Enable)"=FALSE, "VISA resource name"=w413) -> ("error out"=w399:errorcluster, "VISA resource name out"=w412:refnum<visa-resource-name>)  [unwired: 7 in]
        n266 = call <vilib>:"Clear Errors.vi"("error in (no error)"=w399) -> ("error out"=w404:errorcluster)  [unwired: 5 in, 1 out]
        n267 = call "Compile error.vi"("错误输入"=w399) -> ("Error out"=w403:string)  [unwired: 10 in]
        n268 = property on="source" class="Str"("Value"=w403) -> ()  [unwired: 2 in, 2 out]
        n269 = call "FGV_VISA_Comm.vi"("Write?"=TRUE, "error in"=w404, "Host VISA resource name"=w398, "ACC VISA resource name"=w412) -> ()  [unwired: 3 in, 5 out]
        n270 = property on="Status" class="Bool (严格)"("Value"=FALSE ("Status")) -> ()  [unwired: 2 in, 2 out]
      }
      frame "Config_Reset" {
        # "VISA关闭通道、清除保护电路"
        n271 = To Variant(anything=FALSE) -> (Variant=w442:variant)
        n272 = Bundle By Name(cluster=cluster{"Instruct":string, "Data":variant} {"Instruct"="", "Data"=variant}, "Instruct"="Stop", "Data"=w442) -> (w445:cluster{"Instruct":string, "Data":variant})
        n273 = call "FGV_VISA_Comm.vi"() -> ("error out"=w422:errorcluster, "Host VISA resource name out"=w423:refnum<visa-resource-name>, "ACC VISA resource name out"=w448:refnum<visa-resource-name>)  [unwired: 7 in, 2 out]
        n274 = Send Notification(notification=w445, notifier=w441) -> ()  [unwired: 1 in, 2 out]
        n275 = call <userlib>:"Configure OUTPut ENABle.vi"("error in (no error)"=w422, "Enable OUTPut (T: Enable)"=FALSE, "VISA resource name"=w448) -> ("error out"=w438:errorcluster, "VISA resource name out"=w439:refnum<visa-resource-name>)  [unwired: 7 in]
        n276 = call <userlib>:"Configure OUTPut ENABle.vi"("error in (no error)"=w422, "Enable OUTPut (T: Enable)"=FALSE, "VISA resource name"=w423) -> ("error out"=w426:errorcluster, "VISA resource name out"=w425:refnum<visa-resource-name>)  [unwired: 7 in]
        n277 = call <userlib>:"Configure VOLTage PROTection CLEar.vi"("error in (no error)"=w438, "VISA resource name"=w439) -> ("error out"=w436:errorcluster, "VISA resource name out"=w437:refnum<visa-resource-name>)  [unwired: 8 in]
        n278 = call <userlib>:"Configure VOLTage PROTection CLEar.vi"("error in (no error)"=w426, "VISA resource name"=w425) -> ("error out"=w428:errorcluster, "VISA resource name out"=w427:refnum<visa-resource-name>)  [unwired: 8 in]
        n279 = call <userlib>:"Configure CURRent PROTection CLEar.vi"("error in (no error)"=w436, "VISA resource name"=w437) -> ("error out"=w435:errorcluster, "VISA resource name out"=w434:refnum<visa-resource-name>)  [unwired: 8 in]
        n280 = call <userlib>:"Configure CURRent PROTection CLEar.vi"("error in (no error)"=w428, "VISA resource name"=w427) -> ("error out"=w429:errorcluster, "VISA resource name out"=w430:refnum<visa-resource-name>)  [unwired: 8 in]
        n281 = call <userlib>:"Read OUTPut ENABle.vi"("error in (no error)"=w435, "等待时间（毫秒）"=u32 50, "VISA resource name"=w434) -> ("error out"=w416:errorcluster, "OUTPut Status"=w420:bool, "VISA resource name out"=w432:refnum<visa-resource-name>)  [unwired: 6 in]
        n282 = call <userlib>:"Read OUTPut ENABle.vi"("error in (no error)"=w429, "等待时间（毫秒）"=u32 50, "VISA resource name"=w430) -> ("error out"=w415:errorcluster, "OUTPut Status"=w419:bool, "VISA resource name out"=w421:refnum<visa-resource-name>)  [unwired: 6 in]
        n283 = Build Array(w420, w419) -> (w418:bool[])
        n284 = Merge Errors(w416, w415) -> (w414:errorcluster)
        n285 = Or Array Elements(Boolean array=w418) -> (logical OR=w417:bool)
        n286 = property on="On/Off" class="Bool (严格)"("Value"=w417) -> ()  [unwired: 2 in, 2 out]
        n287 = call "FGV_VISA_Comm.vi"("Write?"=TRUE, "error in"=w414, "Host VISA resource name"=w421, "ACC VISA resource name"=w432) -> ()  [unwired: 3 in, 5 out]
      }
      frame "Query_VORTage" {
        w456 = u32 50 ("等待时间（毫秒）")
        w457 = T10."VOLTage" ("VOLTage Tab")
        # "查询当前输出电压值"
        n288 = call "FGV_VISA_Comm.vi"() -> ("error out"=w454:errorcluster, "Host VISA resource name out"=w455:refnum<visa-resource-name>, "ACC VISA resource name out"=w465:refnum<visa-resource-name>)  [unwired: 7 in, 2 out]
        n289 = call <userlib>:"Read VOLTage.vi"("error in (no error)"=w454, "等待时间（毫秒）"=w456, "VOLTage Tab"=w457, "VISA resource name"=w455) -> ("error out"=w451:errorcluster, "VOLTage  Value"=w449:dbl, "VISA resource name out"=w453:refnum<visa-resource-name>)  [unwired: 5 in]
        n290 = call <userlib>:"Read VOLTage.vi"("error in (no error)"=w454, "等待时间（毫秒）"=w456, "VOLTage Tab"=w457, "VISA resource name"=w465) -> ("error out"=w462:errorcluster, "VOLTage  Value"=w464:dbl, "VISA resource name out"=w463:refnum<visa-resource-name>)  [unwired: 5 in]
        n291 = property on="ACC Voltage" class="DigNum (严格)"("Value"=w464) -> ()  [unwired: 2 in, 2 out]
        n292 = property on="Host Voltage" class="DigNum (严格)"("Value"=w449) -> ()  [unwired: 2 in, 2 out]
        n293 = call <userlib>:"Read VOLTage.vi"("error in (no error)"=w462, "等待时间（毫秒）"=u32 50, "VOLTage Tab"=T10."MAXimum", "VISA resource name"=w463) -> ("error out"=w452:errorcluster, "VOLTage  Value"=w458:dbl, "VISA resource name out"=w461:refnum<visa-resource-name>)  [unwired: 5 in]
        n294 = property on="Max voltage" class="DigNum (严格)"("Value"=w458) -> ()  [unwired: 2 in, 2 out]
        n295 = Merge Errors(w452, w451) -> (w450:errorcluster)
        n296 = call "FGV_VISA_Comm.vi"("Write?"=TRUE, "error in"=w450, "Host VISA resource name"=w453, "ACC VISA resource name"=w461) -> ()  [unwired: 3 in, 5 out]
      }
      frame "Query_CURRent" {
        w467 = u32 50 ("等待时间（毫秒）")
        w468 = T12."current" ("Current Tab")
        # "查询当前输出电流值"
        n297 = call "FGV_VISA_Comm.vi"() -> ("error out"=w474:errorcluster, "Host VISA resource name out"=w475:refnum<visa-resource-name>, "ACC VISA resource name out"=w478:refnum<visa-resource-name>)  [unwired: 7 in, 2 out]
        n298 = call <userlib>:"Read CURRent.vi"("error in (no error)"=w474, "等待时间（毫秒）"=w467, "Current Tab"=w468, "VISA resource name"=w478) -> ("error out"=w471:errorcluster, "Current"=w476:dbl, "VISA resource name out"=w477:refnum<visa-resource-name>)  [unwired: 5 in]
        n299 = call <userlib>:"Read CURRent.vi"("error in (no error)"=w474, "等待时间（毫秒）"=w467, "Current Tab"=w468, "VISA resource name"=w475) -> ("error out"=w470:errorcluster, "Current"=w472:dbl, "VISA resource name out"=w473:refnum<visa-resource-name>)  [unwired: 5 in]
        n300 = property on="Host Current" class="DigNum (严格)"("Value"=w472) -> ()  [unwired: 2 in, 2 out]
        n301 = property on="ACC Current" class="DigNum (严格)"("Value"=w476) -> ()  [unwired: 2 in, 2 out]
        n302 = Merge Errors(w471, w470) -> (w469:errorcluster)
        n303 = call "FGV_VISA_Comm.vi"("Write?"=TRUE, "error in"=w469, "Host VISA resource name"=w473, "ACC VISA resource name"=w477) -> ()  [unwired: 3 in, 5 out]
      }
      frame "Query_VOLTage PROTection" {
        w486 = T10."VOLTage" ("VOLTage Tab")
        # "查询当前输出电压保护阀值"
        n304 = call "FGV_VISA_Comm.vi"() -> ("error out"=w485:errorcluster, "Host VISA resource name out"=w487:refnum<visa-resource-name>, "ACC VISA resource name out"=w490:refnum<visa-resource-name>)  [unwired: 7 in, 2 out]
        n305 = call <userlib>:"Read VOLTage PROTection LEVel.vi"("error in (no error)"=w485, "VOLTage Tab"=w486, "VISA resource name"=w490) -> ("error out"=w482:errorcluster, "VOLTage protection level"=w488:dbl, "VISA resource name out"=w489:refnum<visa-resource-name>)  [unwired: 6 in]
        n306 = call <userlib>:"Read VOLTage PROTection LEVel.vi"("error in (no error)"=w485, "VOLTage Tab"=w486, "VISA resource name"=w487) -> ("error out"=w480:errorcluster, "VOLTage protection level"=w483:dbl, "VISA resource name out"=w484:refnum<visa-resource-name>)  [unwired: 6 in]
        n307 = property on="Host OVP" class="DigNum (严格)"("Value"=w483) -> ()  [unwired: 2 in, 2 out]
        n308 = property on="ACC OVP" class="DigNum (严格)"("Value"=w488) -> ()  [unwired: 2 in, 2 out]
        n309 = Merge Errors(w482, w480) -> (w481:errorcluster)
        n310 = call "FGV_VISA_Comm.vi"("Write?"=TRUE, "error in"=w481, "Host VISA resource name"=w484, "ACC VISA resource name"=w489) -> ()  [unwired: 3 in, 5 out]
      }
      frame "Query_CURRent PROTection" {
        w497 = T12."current" ("Current Tab")
        # "查询当前输出电流保护阀值"
        n311 = call "FGV_VISA_Comm.vi"() -> ("error out"=w498:errorcluster, "Host VISA resource name out"=w499:refnum<visa-resource-name>, "ACC VISA resource name out"=w502:refnum<visa-resource-name>)  [unwired: 7 in, 2 out]
        n312 = call <userlib>:"Read CURRent PROTection LEVel.vi"("error in (no error)"=w498, "Current Tab"=w497, "VISA resource name"=w502) -> ("error out"=w495:errorcluster, "Current protection level"=w500:dbl, "VISA resource name out"=w501:refnum<visa-resource-name>)  [unwired: 6 in]
        n313 = call <userlib>:"Read CURRent PROTection LEVel.vi"("error in (no error)"=w498, "Current Tab"=w497, "VISA resource name"=w499) -> ("error out"=w494:errorcluster, "Current protection level"=w492:dbl, "VISA resource name out"=w496:refnum<visa-resource-name>)  [unwired: 6 in]
        n314 = property on="Host OCP" class="DigNum (严格)"("Value"=w492) -> ()  [unwired: 2 in, 2 out]
        n315 = property on="ACC OCP" class="DigNum (严格)"("Value"=w500) -> ()  [unwired: 2 in, 2 out]
        n316 = Merge Errors(w495, w494) -> (w493:errorcluster)
        n317 = call "FGV_VISA_Comm.vi"("Write?"=TRUE, "error in"=w493, "Host VISA resource name"=w496, "ACC VISA resource name"=w501) -> ()  [unwired: 3 in, 5 out]
      }
      frame "Query_VOLTage PROTection ENABle" {
        # "查询当前输出电压保护电路是否使能"
        n318 = call "FGV_VISA_Comm.vi"() -> ("error out"=w509:errorcluster, "Host VISA resource name out"=w510:refnum<visa-resource-name>, "ACC VISA resource name out"=w512:refnum<visa-resource-name>)  [unwired: 7 in, 2 out]
        n319 = call <userlib>:"Read VOLTage PROTection STATus.vi"("error in (no error)"=w509, "VISA resource name"=w512) -> ("error out"=w507:errorcluster, "VOLTage Protection Status"=w511:bool, "VISA resource name out"=w513:refnum<visa-resource-name>)  [unwired: 6 in, 1 out]
        n320 = call <userlib>:"Read VOLTage PROTection STATus.vi"("error in (no error)"=w509, "VISA resource name"=w510) -> ("error out"=w506:errorcluster, "VOLTage Protection Status"=w504:bool, "VISA resource name out"=w508:refnum<visa-resource-name>)  [unwired: 6 in, 1 out]
        n321 = property on="ACCOVPEnable" class="Bool (严格)"("Value"=w511) -> ()  [unwired: 2 in, 2 out]
        n322 = property on="HostOVPEnable" class="Bool (严格)"("Value"=w504) -> ()  [unwired: 2 in, 2 out]
        n323 = Merge Errors(w507, w506) -> (w505:errorcluster)
        n324 = call "FGV_VISA_Comm.vi"("Write?"=TRUE, "error in"=w505, "Host VISA resource name"=w508, "ACC VISA resource name"=w513) -> ()  [unwired: 3 in, 5 out]
      }
      frame "Query_CURRent PROTection ENABle" {
        # "查询当前输出电流保护电路是否使能"
        n325 = call "FGV_VISA_Comm.vi"() -> ("error out"=w520:errorcluster, "Host VISA resource name out"=w521:refnum<visa-resource-name>, "ACC VISA resource name out"=w524:refnum<visa-resource-name>)  [unwired: 7 in, 2 out]
        n326 = call <userlib>:"Read CURRent PROTection STATus.vi"("error in (no error)"=w520, "VISA resource name"=w524) -> ("error out"=w518:errorcluster, "Current Protection Status"=w522:bool, "VISA resource name out"=w523:refnum<visa-resource-name>)  [unwired: 6 in, 1 out]
        n327 = call <userlib>:"Read CURRent PROTection STATus.vi"("error in (no error)"=w520, "VISA resource name"=w521) -> ("error out"=w517:errorcluster, "Current Protection Status"=w515:bool, "VISA resource name out"=w519:refnum<visa-resource-name>)  [unwired: 6 in, 1 out]
        n328 = property on="ACCOCPEnable" class="Bool (严格)"("Value"=w522) -> ()  [unwired: 2 in, 2 out]
        n329 = property on="HostOCPEnable" class="Bool (严格)"("Value"=w515) -> ()  [unwired: 2 in, 2 out]
        n330 = Merge Errors(w518, w517) -> (w516:errorcluster)
        n331 = call "FGV_VISA_Comm.vi"("Write?"=TRUE, "error in"=w516, "Host VISA resource name"=w519, "ACC VISA resource name"=w523) -> ()  [unwired: 3 in, 5 out]
      }
      frame "Query_OUTPut" {
        w536 = u32 50 ("等待时间（毫秒）")
        # "查询通道输出状态"
        n332 = call "FGV_VISA_Comm.vi"() -> ("error out"=w534:errorcluster, "Host VISA resource name out"=w535:refnum<visa-resource-name>, "ACC VISA resource name out"=w538:refnum<visa-resource-name>)  [unwired: 7 in, 2 out]
        n333 = call <userlib>:"Read OUTPut ENABle.vi"("error in (no error)"=w534, "等待时间（毫秒）"=w536, "VISA resource name"=w538) -> ("error out"=w532:errorcluster, "OUTPut Status"=w529:bool, "VISA resource name out"=w537:refnum<visa-resource-name>)  [unwired: 6 in]
        n334 = call <userlib>:"Read OUTPut ENABle.vi"("error in (no error)"=w534, "等待时间（毫秒）"=w536, "VISA resource name"=w535) -> ("error out"=w531:errorcluster, "OUTPut Status"=w528:bool, "VISA resource name out"=w533:refnum<visa-resource-name>)  [unwired: 6 in]
        n335 = Build Array(w529, w528) -> (w527:bool[])
        n336 = Merge Errors(w532, w531) -> (w530:errorcluster)
        n337 = Or Array Elements(Boolean array=w527) -> (logical OR=w526:bool)
        n338 = property on="On/Off" class="Bool (严格)"("Value"=w526) -> ()  [unwired: 2 in, 2 out]
        n339 = call "FGV_VISA_Comm.vi"("Write?"=TRUE, "error in"=w530, "Host VISA resource name"=w533, "ACC VISA resource name"=w537) -> ()  [unwired: 3 in, 5 out]
      }
      frame "Exit" {
        # "退出"
        n340 = To Variant(anything=FALSE) -> (Variant=w549:variant)
        n341 = Bundle By Name(cluster=cluster{"Instruct":string, "Data":variant} {"Instruct"="", "Data"=variant} ("通知"), "Instruct"="Exit", "Data"=w549) -> (w552:cluster{"Instruct":string, "Data":variant})
        n342 = Send Notification(notification=w552, notifier=w548) -> ()  [unwired: 1 in, 2 out]
        n343 = property on="ExecuteTime(s)" class="DigNum (严格)"() -> ("Value"=w547:dbl)  [unwired: 2 in, 2 out]
        n344 = property on="Pause up(ms)" class="DigNum (严格)"() -> ("Value"=w546:dbl)  [unwired: 2 in, 2 out]
        n345 = property on="Pause next(ms)" class="DigNum (严格)"() -> ("Value"=w540:dbl)  [unwired: 2 in, 2 out]
        n346 = Build Array(w547, w546, w540) -> (w545:dbl[])
        n347 = Flatten To XML(6:w545) -> (2:w544:string)
        n348 = call "Examine Path.vi"("Filename"="MianData.xml") -> ("error out"=w543:errorcluster, "Path"=w542:path)  [unwired: 9 in]
        n349 = call-poly <vilib>:"Write to XML File.vi"("error in (no error)"=w543, "XML Input"=w544, "XML File Path"=w542) -> ()  [unwired: 6 in, 3 out]
      }
    }
  }
  n350 = while {
    tunnel: w27 -> [_]
    stop <- w558 stop-if-true
    n351 = event shown="[0] 超时" {
      selector: _ -> [_ _ _ _ _ _ _ _ _ _ _ _ _ _]
      dyn-events: _ -> [_ _ _ _ _ _ _ _ _ _ _ _ _ _]
      timeout: 5 -> [_ _ _ _ _ _ _ _ _ _ _ _ _ _]
      tunnel: [w572 w603 string[] ["Config_Reset"] ("Instruct") string[] ["VISA_Close", "VISA_Config", "VISA_Open", "Config_Off", "Query_OUTPut", "Query_VORTage", "Query_CURRent", "Query_VOLTage PROTection", "Query_CURRent PROTection", "Query_VOLTage PROTection ENABle", "Query_CURRent PROTection ENABle"] ("Instruct") string[] ["PCAN_Close", "PCAN_Config", "PCAN_Open"] ("Instruct") string[] ["Transmit_info"] ("Instruct") string[] ["Config_VOLTage"] ("Instruct") string[] ["Config_CURRent"] ("Instruct") string[] ["Config_VOLTage PROTection"] ("Instruct") string[] ["Config_CURRent PROTection"] ("Instruct") string[] ["Config_VOLTage PROTection ENABle"] ("Instruct") string[] ["Config_CURRent PROTection ENABle"] ("Instruct") _ string[] ["Config_Off", "Config_VOLTage", "VISA_Close", "PCAN_Close", "Exit"] ("Instruct")] -> w560
      tunnel: [_ _ _ _ _ _ _ _ _ _ _ _ _ variant[] [] ("Data")] -> w559
      tunnel: [_ _ _ _ _ _ _ _ _ _ _ _ _ TRUE] -> w558
      event Timeout {
        n352 = event-data() -> ()  [unwired: 1 in, 3 out]
        n353 = property on="ACC Voltage" class="DigNum (严格)"() -> ("Value"=w563:dbl)  [unwired: 2 in, 2 out]
        n354 = property on="Max voltage" class="DigNum (严格)"() -> ("Value"=w568:dbl)  [unwired: 2 in, 2 out]
        n355 = property on="On/Off" class="Bool (严格)"() -> ("Value"=w564:bool)  [unwired: 2 in, 2 out]
        n356 = property on="Pause up(ms)" class="DigNum (严格)"() -> ("Value"=w566:dbl)  [unwired: 2 in, 2 out]
        n357 = Not Equal To 0?(x=w566) -> (x != 0?=w565:bool)
        n358 = Less Or Equal?(x=w563, y=w568) -> (x <= y?=w567:bool)
        n359 = feedback-in #2(w564) -> ()
        n360 = feedback #2(FALSE ("Value")) -> (w571:bool)
        n361 = Compound Arithmetic op=AND ("复合运算")(w564, w567, w565) -> (w569:bool)
        n362 = case shown="真" w569 {
          tunnel: [w574 w589] -> w572
          tunnel: w571 -> [_ w588]
          tunnel: w564 -> [_ _]
          frame False {
            n363 = case shown="假" FALSE {
              tunnel: [_ string[] ["Save record", "Config_Off", "Config_VOLTage", "Query_OUTPut", "Fool-proof"] ("Instruct")] -> w574
              frame False {
              }
              frame True {
              }
            }
          }
          frame True {
            n364 = Not(x=w588) -> (.not. x?=w577:bool)
            n365 = feedback #3(FALSE ("Time has Elapsed")) -> (w578:bool)
            n366 = Or(x=w577, y=w578) -> (x .or. y?=w576:bool)
            n367 = call "Random.vi"("Write?"=w576, "lower bound(ms)"="Pause next(ms)", "upper bound(ms)"="Pause up(ms)", "ExecuteTime(s)"="ExecuteTime(s)") -> ("Time Target (s)"=w584:dbl)  [unwired: 7 in]
            n368 = call "已用时间"("Time Target (s)"=w584, "Reset"=w577) -> ("Elapsed Time (s)"=w586:dbl, "Time has Elapsed"=w580:bool)  [unwired: 10 in, 6 out]
            n369 = feedback-in #3(w580) -> ()
            n370 = Add(x="ExecuteTime(s)", y=0.5) -> (x+y=w585:dbl)
            n371 = case shown="假" w580 {
              tunnel: [w596 string[] ["Config_On ACC"] ("Instruct")] -> w589
              tunnel: w586 -> [w598 _]
              tunnel: w577 -> [w594 _]
              tunnel: "ExecuteTime(s)" -> [w592 _]
              tunnel: w585 -> [w591 _]
              frame False {
                n372 = Greater?(x=w598, y=w591) -> (0:w595:bool)
                n373 = Or(x=w595, y=w594) -> (x .or. y?=w593:bool)
                n374 = call "已用时间2"("Time Target (s)"=w592, "Reset"=w593) -> ("Elapsed Time (s)"=→"Elapsed Time (s)":dbl, "Time has Elapsed"=w597:bool)  [unwired: 10 in, 6 out]
                n375 = case shown="真" w597 {
                  tunnel: [_ string[] ["record", "Config_Off ACC"] ("Instruct")] -> w596
                  frame False {
                  }
                  frame True {
                  }
                }
              }
              frame True {
              }
            }
          }
        }
      }
      event "On/Off": Value Change {
        n376 = event-data() -> ("NewVal"=w602:bool)  [unwired: 1 in, 5 out]
        n377 = Select(t=string[] ["Fool-proof", "Config_VOLTage", "Config_CURRent", "Config_On"] ("Instruct"), s=w602, f=string[] ["Config_Off", "Save record", "Config_VOLTage", "Config_CURRent", "Fool-proof"] ("Instruct")) -> (s? t:f=w603:string[])
        n378 = case shown="真" w602 {
          tunnel: ["Await the opportune moment" "Begin testing"] -> w601
          frame False {
          }
          frame True {
            n379 = property on="List record" class="MCListbox (严格)"("ItemNames"=string[][] [] ("项名")) -> ()  [unwired: 2 in, 2 out]
          }
        }
        n380 = property on="Status:" class="Str"("Value"=w601) -> ()  [unwired: 2 in, 2 out]
      }
      event "Reset": Value Change {
        n381 = event-data() -> ()  [unwired: 1 in, 6 out]
        n382 = property on="Status:" class="Str"("Value"="Reset") -> ()  [unwired: 2 in, 2 out]
      }
      event "RS232 Config": Value Change {
        n383 = event-data() -> ()  [unwired: 1 in, 6 out]
        n384 = property on="Status:" class="Str"("Value"="RS232 Config") -> ()  [unwired: 2 in, 2 out]
      }
      event "PCAN Config": Value Change {
        n385 = event-data() -> ()  [unwired: 1 in, 6 out]
        n386 = property on="Status:" class="Str"("Value"="PCAN Config") -> ()  [unwired: 2 in, 2 out]
      }
      event "Transmit info": Value Change {
        n387 = event-data() -> ()  [unwired: 1 in, 6 out]
        n388 = property on="Status:" class="Str"("Value"="Transmit info") -> ()  [unwired: 2 in, 2 out]
      }
      event "ACC Voltage", "Host Voltage": Value Change {
        n389 = event-data() -> ()  [unwired: 1 in, 6 out]
      }
      event "ACC Current", "Host Current": Value Change {
        n390 = event-data() -> ()  [unwired: 1 in, 6 out]
      }
      event "ACC OVP", "Host OVP": Value Change {
        n391 = event-data() -> ()  [unwired: 1 in, 6 out]
      }
      event "ACC OCP", "Host OCP": Value Change {
        n392 = event-data() -> ()  [unwired: 1 in, 6 out]
      }
      event "ACCOVPEnable", "HostOVPEnable": Value Change {
        n393 = event-data() -> ()  [unwired: 1 in, 6 out]
      }
      event "ACCOCPEnable", "HostOCPEnable": Value Change {
        n394 = event-data() -> ()  [unwired: 1 in, 6 out]
      }
      event "Receive": Mouse Down {
        n395 = event-data() -> ("CtlRef"=w626:refnum<vi>, "Coords"=w625:T13)  [unwired: 1 in, 6 out]
        n396 = invoke class="MCListbox (严格)" method="Point To Row Column"(reference=w626, "Point"=w625) -> ("CellPosition"=w624:T14)  [unwired: 5 in, 6 out]
        n397 = Unbundle By Name(w624) -> ("Row"=w623:i32)
        n398 = property on="Receive" class="MCListbox (严格)"("Value"=w623) -> ()  [unwired: 2 in, 2 out]
      }
      event Panel Close? {
        n399 = event-data() -> ()  [unwired: 1 in, 4 out]
        n400 = property on="Status:" class="Str"("Value"="Exit") -> ()  [unwired: 2 in, 2 out]
        n401 = event-data("Discard?"=TRUE ("放弃？")) -> ()  [unwired: 1 in, 1 out]
      }
    }
    n402 = Format Date/Time String(time format string (%c)="%Y/%m/%d %H:%M:%S" ("时间格式字符串(%c)")) -> (date/time string=→"Time:":string)  [unwired: 2 in]
    n403 = call "Queue.vi"("State"=QueueState."In", "Data"=w559, "Instruct"=w560) -> ()  [unwired: 6 in, 3 out]
    "Company:" <- "Hinge-teck" ("Company:")
  }
  n404 = while {
    tunnel: w20 -> [w633]
    tunnel: w18 -> [w647]
    shift-right: [w638] -> _
    shift-left: "" ("Instruct") -> [w644]
    shift-right: [w637] -> _
    shift-left: FALSE -> [w639]
    tunnel: w19 -> [w634]
    tunnel: [w634] -> w8
    tunnel: [w633] -> w16
    stop <- w636 stop-if-true
    w632 = 10 ("超时毫秒(-1)")
    # "PCAN Write"
    n405 = Wait on Notification(notifier=w647, timeout in ms (-1)=w632, error in (no error)=w633) -> (notification=w646:cluster{"Instruct":string, "Data":variant})  [unwired: 1 in, 3 out]
    n406 = Unbundle By Name(w646) -> ("Instruct"=w645:string, "Data"=w642:variant)
    n407 = Variant To Data(type=FALSE, Variant=w642) -> (data=w640:bool, error out=w635:errorcluster)  [unwired: 1 in]
    n408 = Empty String/Path?(string/path=w645) -> (empty?=w643:bool)
    n409 = Select(t=w644, s=w643, f=w645) -> (s? t:f=w638:string)
    n410 = call <vilib>:"Clear Errors.vi"("error in (no error)"=w635) -> ()  [unwired: 5 in, 2 out]
    n411 = Select(t=w639, s=w643, f=w640) -> (s? t:f=w637:bool)
    n412 = case shown="\"Start\"" w638 {
      tunnel: w637 -> [_ _ _]
      tunnel: [_ _ TRUE] -> w636
      tunnel: w634 -> [_ w652 _]
      tunnel: w632 -> [_ w648 _]
      frame "假", Default {
      }
      frame "Start" {
        n413 = Dequeue Element(queue=w652, timeout in ms (-1)=w648) -> (element=w651:cluster{"instruct":string, "data":variant})  [unwired: 1 in, 3 out]
        n414 = Unbundle By Name(w651) -> ("instruct"=w650:string, "data"=w649:variant)
        n415 = case shown="\"PCAN_Write\"" w650 {
          tunnel: w649 -> [_ w659]
          frame "假", Default {
          }
          frame "PCAN_Write" {
            n416 = Tick Count (ms)() -> (millisecond timer value=w654:u32)
            n417 = feedback-in #4(w654) -> ()
            n418 = feedback #4() -> (w653:u32)  [unwired: 1 in]
            n419 = Subtract(x=w654, y=w653) -> (x-y=→"x-y":u32)
            n420 = Variant To Data(type=T15 [] ("MessageBuffer"), Variant=w659) -> (data=w657:T15)  [unwired: 1 in, 1 out]
            n421 = call "FGV_PCAN_Config.vi"() -> ("Channel out"=w656:T1)  [unwired: 8 in, 3 out]
            n422 = for {
              tunnel: w657 -> [w660] mode=indexing
              tunnel: w656 -> [w661]
              tunnel: [w660] -> _ mode=indexing
              n423 = call <userlib>:"CAN Write.vi"("Channel"=w661, "MessageBuffer"=w660) -> ()  [unwired: 2 out]
            }
          }
        }
      }
      frame "Exit" {
      }
    }
  }
  n424 = while {
    tunnel: w19 -> [w683]
    tunnel: w6 -> [w682]
    tunnel: w20 -> [w667]
    tunnel: w18 -> [w679]
    shift-right: [w669] -> _
    shift-left: "" ("Instruct") -> [w672]
    shift-right: [w671] -> _
    shift-left: FALSE -> [w670]
    tunnel: [w667] -> w17
    stop <- w668 stop-if-true
    n425 = property on="LastError" class="Str"() -> ("Value"=w664:string)  [unwired: 2 in, 2 out]
    n426 = Wait on Notification(notifier=w679, timeout in ms (-1)=10 ("超时毫秒(-1)"), error in (no error)=w667) -> (notification=w680:cluster{"Instruct":string, "Data":variant})  [unwired: 1 in, 3 out]
    n427 = Unbundle By Name(w680) -> ("Instruct"=w673:string, "Data"=w674:variant)
    n428 = Variant To Data(type=FALSE, Variant=w674) -> (data=w676:bool, error out=w675:errorcluster)  [unwired: 1 in]
    n429 = call "Connect error.vi"("LastError"=w664, "PCAN Read error"="PCAN Read error", "source"="source") -> ("LastError out"=→"LastError":string)  [unwired: 8 in]
    n430 = Empty String/Path?(string/path=w673) -> (empty?=w678:bool)
    n431 = call <vilib>:"Clear Errors.vi"("error in (no error)"=w675) -> ()  [unwired: 5 in, 2 out]
    n432 = Select(t=w672, s=w678, f=w673) -> (s? t:f=w669:string)
    n433 = Select(t=w670, s=w678, f=w676) -> (s? t:f=w671:bool)
    n434 = case shown="\"Start\"" w669 {
      tunnel: w683 -> [_ w689 _]
      tunnel: w682 -> [_ w688 _]
      tunnel: [_ _ TRUE] -> w668
      frame "假", Default {
      }
      frame "Start" {
        n435 = call "Conformity.vi"() -> ("整合后"=w686:T16, "时间段"=w685:u16[])  [unwired: 10 in]
        n436 = call "Timing.vi"("数组"=w685) -> ("当前"=w687:u16, "到"=w684:bool)  [unwired: 8 in, 1 out]
        n437 = case shown="真" w684 {
          tunnel: w689 -> [_ w691]
          tunnel: w688 -> [_ w690]
          tunnel: w687 -> [_ w693]
          tunnel: w686 -> [_ w692]
          frame False {
          }
          frame True {
            n438 = for {
              tunnel: w692 -> [w700] mode=indexing
              tunnel: w693 -> [w698]
              tunnel: w691 -> [w695]
              tunnel: w690 -> [w694]
              n439 = Unbundle By Name(w700) -> ("Time"=w699:u16, "MessageBuffer"=w696:T15)
              n440 = Equal?(x=w698, y=w699) -> (x = y?=w697:bool)
              n441 = case shown="真" w697 {
                tunnel: w696 -> [_ w706]
                tunnel: w695 -> [_ w705]
                tunnel: w694 -> [_ w704]
                frame False {
                }
                frame True {
                  n442 = To Variant(anything=w706) -> (Variant=w701:variant)
                  n443 = Bundle By Name(cluster=cluster{"instruct":string, "data":variant} {"instruct"="PCAN_Write", "data"=variant}, "data"=w701) -> (w703:cluster{"instruct":string, "data":variant})
                  n444 = Enqueue Element(queue=w705, element=w703, error in (no error)=w704) -> ()  [unwired: 1 in, 3 out]
                }
              }
            }
          }
        }
      }
      frame "Exit" {
      }
    }
  }
  n445 = Release Queue(queue=w8) -> ()  [unwired: 2 in, 3 out]
  n446 = Merge Errors(w14, w16, w17) -> (w13:errorcluster)
  n447 = control-ref of="本VI"() -> (w2:refnum<vi>)
  n448 = Release Notifier(notifier=w12, error in (no error)=w13) -> (error out=w1:errorcluster)  [unwired: 1 in, 2 out]
  n449 = disable-structure shown="禁用" {
    disable-tunnel: w2 -> [w709 _]
    disable-tunnel: w1 -> [w708 _]
    frame Disabled {
      n450 = invoke class="VI" method="FP.Close"(reference=w709, error in=w708) -> ()  [unwired: 1 in, 3 out]
    }
    frame Enabled {
    }
  }
  n451 = call "Queue.vi"("State"=QueueState."Close", "error in"=w22) -> ()  [unwired: 7 in, 3 out]
